vi "Main PC Station.vi"() -> ()   [LabVIEW 2015]
uses:
  ramki konfiguracyjne.ctl
  wyj manip.ctl
  wyj auto.ctl
  klapki.ctl
  szablon odometry_filtered_local.ctl
  QMH Fundamentals - Message Cluster.ctl
  CANFrameControl.ctl
  safety_ctl.ctl
  <vilib>/Utility/inputDevices.llb/closeJoystick.vi
  Gobal for ROS.vi
  Global GPS.vi
  <vilib>/MediaMongrels Ltd/WebSockets/WebSockets/WebSockets.lvlib
panel:
  out "szablon VELOCITIES 3":T1
  in  "szablon VELOCITIES 2":T1
  in  "Vlin multiply":dbl
  out "STEERING out":T2
  in  "STEERING":T2
  in  "LABVIEW AUTONOMY DATA":T3={"linear"=0.0, "angular"=0.0, "lin div"=1.0, "ang div"=1.0} {"angular" format="%#_13g"; "linear" format="%#_13g"}
  in  "LV/ROS":enum16{"LABVIEW", "ROS"}(ring)
  in  "szablon odometry/filtered/local":T4
  out "CMD_VEL out":T5
  in  "szablon ARM DRIVE":T6
  out "diody wyj":T7
  in  "szablon VELOCITIES":T1
  in  "klawiatura":bool
  in  "szukaj joy":bool=TRUE
  in  "wyszukaj\nxbox":bool=TRUE
  out "zakresy":cluster{"zak2":bool, "zak1":bool}
  out "MANIPULATOR wy 2":T8
  in  "path":path=path "C:/Users/Kacper/Desktop/Raptorv4/LOGI PREDKOSCI"
  in  "LOG?":bool
  out "RAW NAPEDY":T9
  in  "AUTO":bool
  in  "szablon CMD_VEL":T5
  in  "ster zadane":cluster{dbl, dbl}
  in  "TRIGGER":bool
  out "diody":T10
  in  "path to JPEG file":path=path "C:/Users/Kacper/Downloads/14331560_1175035659222212_341556152_n.png"
  in  "wlacz manipulator":bool
  out "kluster sterowan probnik":T11={"SERWO 6"=127, "SERWO 5"=127, "SERWO 4"=127, "SERWO 3"=127, "ON/OFF Wiertło"=FALSE, "Wiertło PWM"=128, "Wózek PWM"=128, "Stop głębokość"=TRUE, "Głębokość PWM"=128, "speed wózek"=0, "Wózek up"=FALSE, "Wózek down"=FALSE, "Stop wózek"=FALSE, "PROBNK ID 4"=3}
  in  "Zresetuj monitor":bool
  in  "Przestarzała data":bool
  in  "RESET STM":bool
  in  "STOP ??":bool
  out "speed out":cluster{i16, i16, i16, i16, i16, i16} {"?" scale=-32767.0..32767.0; "?" scale=-32767.0..32767.0; "?" scale=-32767.0..32767.0; "?" scale=-32767.0..32767.0; "?" scale=-32767.0..32767.0; "?" scale=-32767.0..32767.0}
  in  "E-Stop":bool
  out "srednie":T12(graph)
  out "UDP connection":bool
  in  "Tab Control 2":enum32{"CAN", "FPGA H&S", "SAFETY"}(tab)
  in  "Tab Control":T13(tab)
  out "Digital Waveform Graph":digitalwaveform(graph)
  out "Mixed Signal Graph":T14(graph)
  in  "STM Prawy ID CAN 2":u32=1
  in  "STM Lewy ID CAN 1":u32=2
  in  "IDD PREDKOSCI 1":u8=1
  in  "IDD PREDKOSCI  2":u8=1
  in  "PRZOD L":T15={"Prąd"=20.0, "Kp"=8.0, "Ki"=3.0, "OK Button"=FALSE, "ID CAN"=2, "IDD"=2, "Sat"=250} {"Ki" format="%.1f"; "Kp" format="%.1f"; "Prąd" format="%.1f"}
  in  "TYL L":T15={"Prąd"=20.0, "Kp"=8.0, "Ki"=3.0, "OK Button"=FALSE, "ID CAN"=2, "IDD"=3, "Sat"=250} {"Ki" format="%.1f"; "Kp" format="%.1f"; "Prąd" format="%.1f"}
  in  "SRODEK L":T15={"Prąd"=20.0, "Kp"=8.0, "Ki"=3.0, "OK Button"=FALSE, "ID CAN"=2, "IDD"=4, "Sat"=250} {"Ki" format="%.1f"; "Kp" format="%.1f"; "Prąd" format="%.1f"}
  in  "SRODEK P":T15={"Prąd"=20.0, "Kp"=8.0, "Ki"=3.0, "OK Button"=FALSE, "ID CAN"=1, "IDD"=4, "Sat"=250} {"Ki" format="%.1f"; "Kp" format="%.1f"; "Prąd" format="%.1f"}
  in  "TYL P":T15={"Prąd"=20.0, "Kp"=8.0, "Ki"=3.0, "OK Button"=FALSE, "ID CAN"=1, "IDD"=3, "Sat"=250} {"Ki" format="%.1f"; "Kp" format="%.1f"; "Prąd" format="%.1f"}
  in  "PRZOD P":T15={"Prąd"=20.0, "Kp"=8.0, "Ki"=3.0, "OK Button"=FALSE, "ID CAN"=1, "IDD"=2, "Sat"=250} {"Ki" format="%.1f"; "Kp" format="%.1f"; "Prąd" format="%.1f"}
  in  "wagi":T16={"l przod"=1.0, "l tyl"=1.0, "l srodek"=1.0, "p przod"=1.0, "p tyl"=1.0, "p srodek"=1.0} {"l przod" format="%#.6g"}
  in  "advertise msg":string="{\"op\":\"advertise\", \"topic\":\"pc/odom\",\"type\":\"sterowanie/velocities\"}"
  in  "rosbridge port":u16=9090
  in  "rosbridge server IP":string="192.168.1.117"
  in  "STOP ROS WRITE":bool
  out "raw frame":string
  in  "Topic to write":string="rio/odom"
  in  "ROSB WRITE":bool
  out "error out":errorcluster
  in  "ROSB READ":bool
  in  "stop 2":bool
  out "Opcode 2":u8
  out "Data 2":string
  in  "rosbridge server IP 2":string="192.168.164.128"
  in  "rosbridge port 2":u16=9090
  in  "error in (no error) 2":errorcluster
  out "error out 3":errorcluster
  in  "Topic to subscribe 2":string="/"
  out "Wykres manipulator":T17(graph)
  in  "Wej manip":T19={"MANIPULATOR ID 3 "=3, "0 bajt"=0, "serwa i pompa"={"4"=TRUE, "1 "=TRUE, "3"=TRUE, "2"=TRUE, "lewy"=TRUE, "serwo 3"=TRUE, "serwo 4 "=TRUE, "przekaznik"=TRUE}}
  in  "ster  manual manipulator":T20 {"DRUGIE 2" scale=0.0..255.0; "PIERWSZE 1" scale=0.0..255.0; "OBROT 0" scale=0.0..255.0; "OBROT 5" scale=0.0..255.0; "CHWYTAK 4" scale=0.0..255.0; "POCHYL 3" scale=0.0..255.0}
  in  "manual/wysylanie":bool
  out "MANIPULATOR wy":T17
  in  "Zbiornik 2":u8(slide)=128 scale=0.0..255.0
  in  "Stop zbiorniki 2":bool
  in  "Zbiornik":u8(slide)=128 scale=70.0..180.0
  in  "pojrmniki 6":u8(slide)=127 scale=0.0..255.0
  in  "SERWO 5":u8(slide)=127 scale=0.0..255.0
  in  "SERWO 4":u8(slide)=127 scale=0.0..255.0
  in  "chwytak 3":u8(slide)=127 scale=0.0..255.0
  in  "Stop głębokość":bool
  in  "Stop wózek":bool
  in  "Wiertło PWM":u8(slide)=128 scale=0.0..255.0
  in  "Gkebokość PWM":u8(slide)=128 scale=0.0..255.0
  in  "Wózek PWM":u8(slide)=128 caption="Vertical Pointer Slide" scale=0.0..255.0
  in  "ON/OFF Wiertło":bool
  in  "speed głębokość":u8
  in  "speed wózek":u8
  out "krańcówka 4":bool
  out "krańcówka 3":bool
  out "krańcówka 2":bool
  out "krańcówka":bool
  in  "PROBNK ID 4":u32=3
  in  "Wózek up":bool
  in  "Głębokość down":bool
  in  "Głębokość up":bool
  in  "Wózek down":bool
  in  "sterowanie joyem probe":bool
  in  "Stop zbiorniki":bool
  out "wiatr":T21 {"prędkosc wiatru km/h" scale=0.0..50.0}
  out "temp/wilg":T22
  out "zap/kierunek":T23
  out "pH":cluster{"temp. pkt rosy":sgl, "pH":sgl}
  in  "ROLL 1":dbl(slide) scale=0.0..1.0
  in  "YAW 1":dbl(slide) scale=0.0..1.0
  in  "PITCH 1":dbl(slide) scale=0.0..1.0
  in  "ile metrow ma przejechac ?":dbl=500.0
  out "teta":dbl
  out "Y":dbl
  out "X":dbl
  out "Location":cluster{"Y":dbl[], "Y":dbl[]}[](graph)
  in  "resset":bool
  in  "Xo":dbl
  in  "Yo":dbl=5.0
  in  "teta pocz.":dbl=90.0
  out "Yaw":dbl
  out "po korekcie":dbl
  out "pozycje z IMU":cluster{"Yaw":dbl, "Pitch":dbl, "Roll":dbl}(graph)
  in  "laser , obiekt ?":bool
  out "przejechane ?":bool
  out "obiekt?":bool
  in  "auto":T24={"zadany"=timestamp(0 s since 1904-01-01), "Autonomia ?"=FALSE, "Time Target (s)"=99999.0, "Reset"=FALSE, "odblokuj timer"=FALSE, "obiekt?"=FALSE, "przejechane ? "=FALSE} {"zadany" format="%<%H:%M:%S\n%x>T"}
  out "wyj auto":T25
  out "GPS Data":T26 {"Fix Quality" items=["Invalid", "GPS Fix", "DGPS Fix", "PPS Fix", "Real Time Kinematic", "Float RTK", "Estimated", "Manual Input Mode", "Simulation Mode"]}
  out "Frames":string[][](table)
  in  "Widocznosc ramek":bool=TRUE
  out "okres [ms]":dbl format="%.3g"
  out "ilosc mesagy":dbl
  in  "Prędkosci Prawy [4]":bool
  in  "Prędkości Lewy [5]":bool
  in  "manipulator [32]":bool
  out "wyj nowe L ?":cluster{"9":sgl, "10":sgl, "8":sgl}
  out "wyj nowe P ? 2":cluster{"9":sgl, "10":sgl, "8":sgl}
  in  "okres watchdoga":u32=100
  in  "wlacz watchdoga":bool
  out "temperatura":sgl(slide) scale=25.0..70.0
  in  "Total (%)":dbl(knob) scale=0.0..100.0
  in  "System Reset":bool
  out "kolejka odbior":i32
  out "kolejka wysylanie":i32
  in  "udp to sbrio":bool
  in  "eventy stop":bool
  out "send ind":i32
  in  "stop queue":bool
  out "receive ind":i32
  in  "UDP odbior in":bool
  in  "stop all":bool
  in  "UDP from sb 2":bool=TRUE
  in  "UDP to sb 2":bool=TRUE
  out "eventy ind":i32
  out "send loop":i32
  out "reciev lloop":i32
  out "safety":i32
  out "lok":i32
  out "lok1":i32
  out "jazda":i32
  out "mani":i32
  out "can":i32
  out "stope health":bool
  out "stope event":bool
  out "stope lokal":bool
  out "stope manip":bool
  out "stope jazda":bool
  out "stope lokal 2":bool
  out "stope odbior":bool
  out "stope wysyl":bool
  out "stope can":bool=TRUE
  out "# pending insert":i32
  out "# pending remove":i32
  in  "index joya\n jazda":i32
  in  "device index":i32=4
  out "wysylanie":bool
  out "graph drazki":cluster{i32[], i32[]}[](graph)
  out "ster. wyj. manipulator":T27
  out "Blokada jazda":bool
  out "graph 1":cluster{i32[], i32[]}[](graph)
  in  "max pwm skrecanie":dbl(slide)=0.5 scale=0.0..1.0
  in  "max pwm przod":dbl(slide)=0.5 min=0.0 max=255.0 scale=0.0..1.0
  out "Wysylanie jazda":bool
  # "max rotation +"
  # "max speed +"
  # "max rotation -"
  # "max speed -"
  # "Os Y +"
  # "Os X +"
  # "trigger"
  # "pitch grip"
  # "PWM 3 os Y\nPWM 4 os X\nPWM 5 T"
  # "gimbal 1"
  # "grip O/Z"
  # "gimbal 2"
  # "roll grip"
  # "Os Y+"
  # "ramie 1"
  # "PWM1 os X \nPWM2 os Y\nPWM 6 T"
  # "ramie 2"
  # "PWM 7 T"
  # "obrot base"
  # "Os X +"
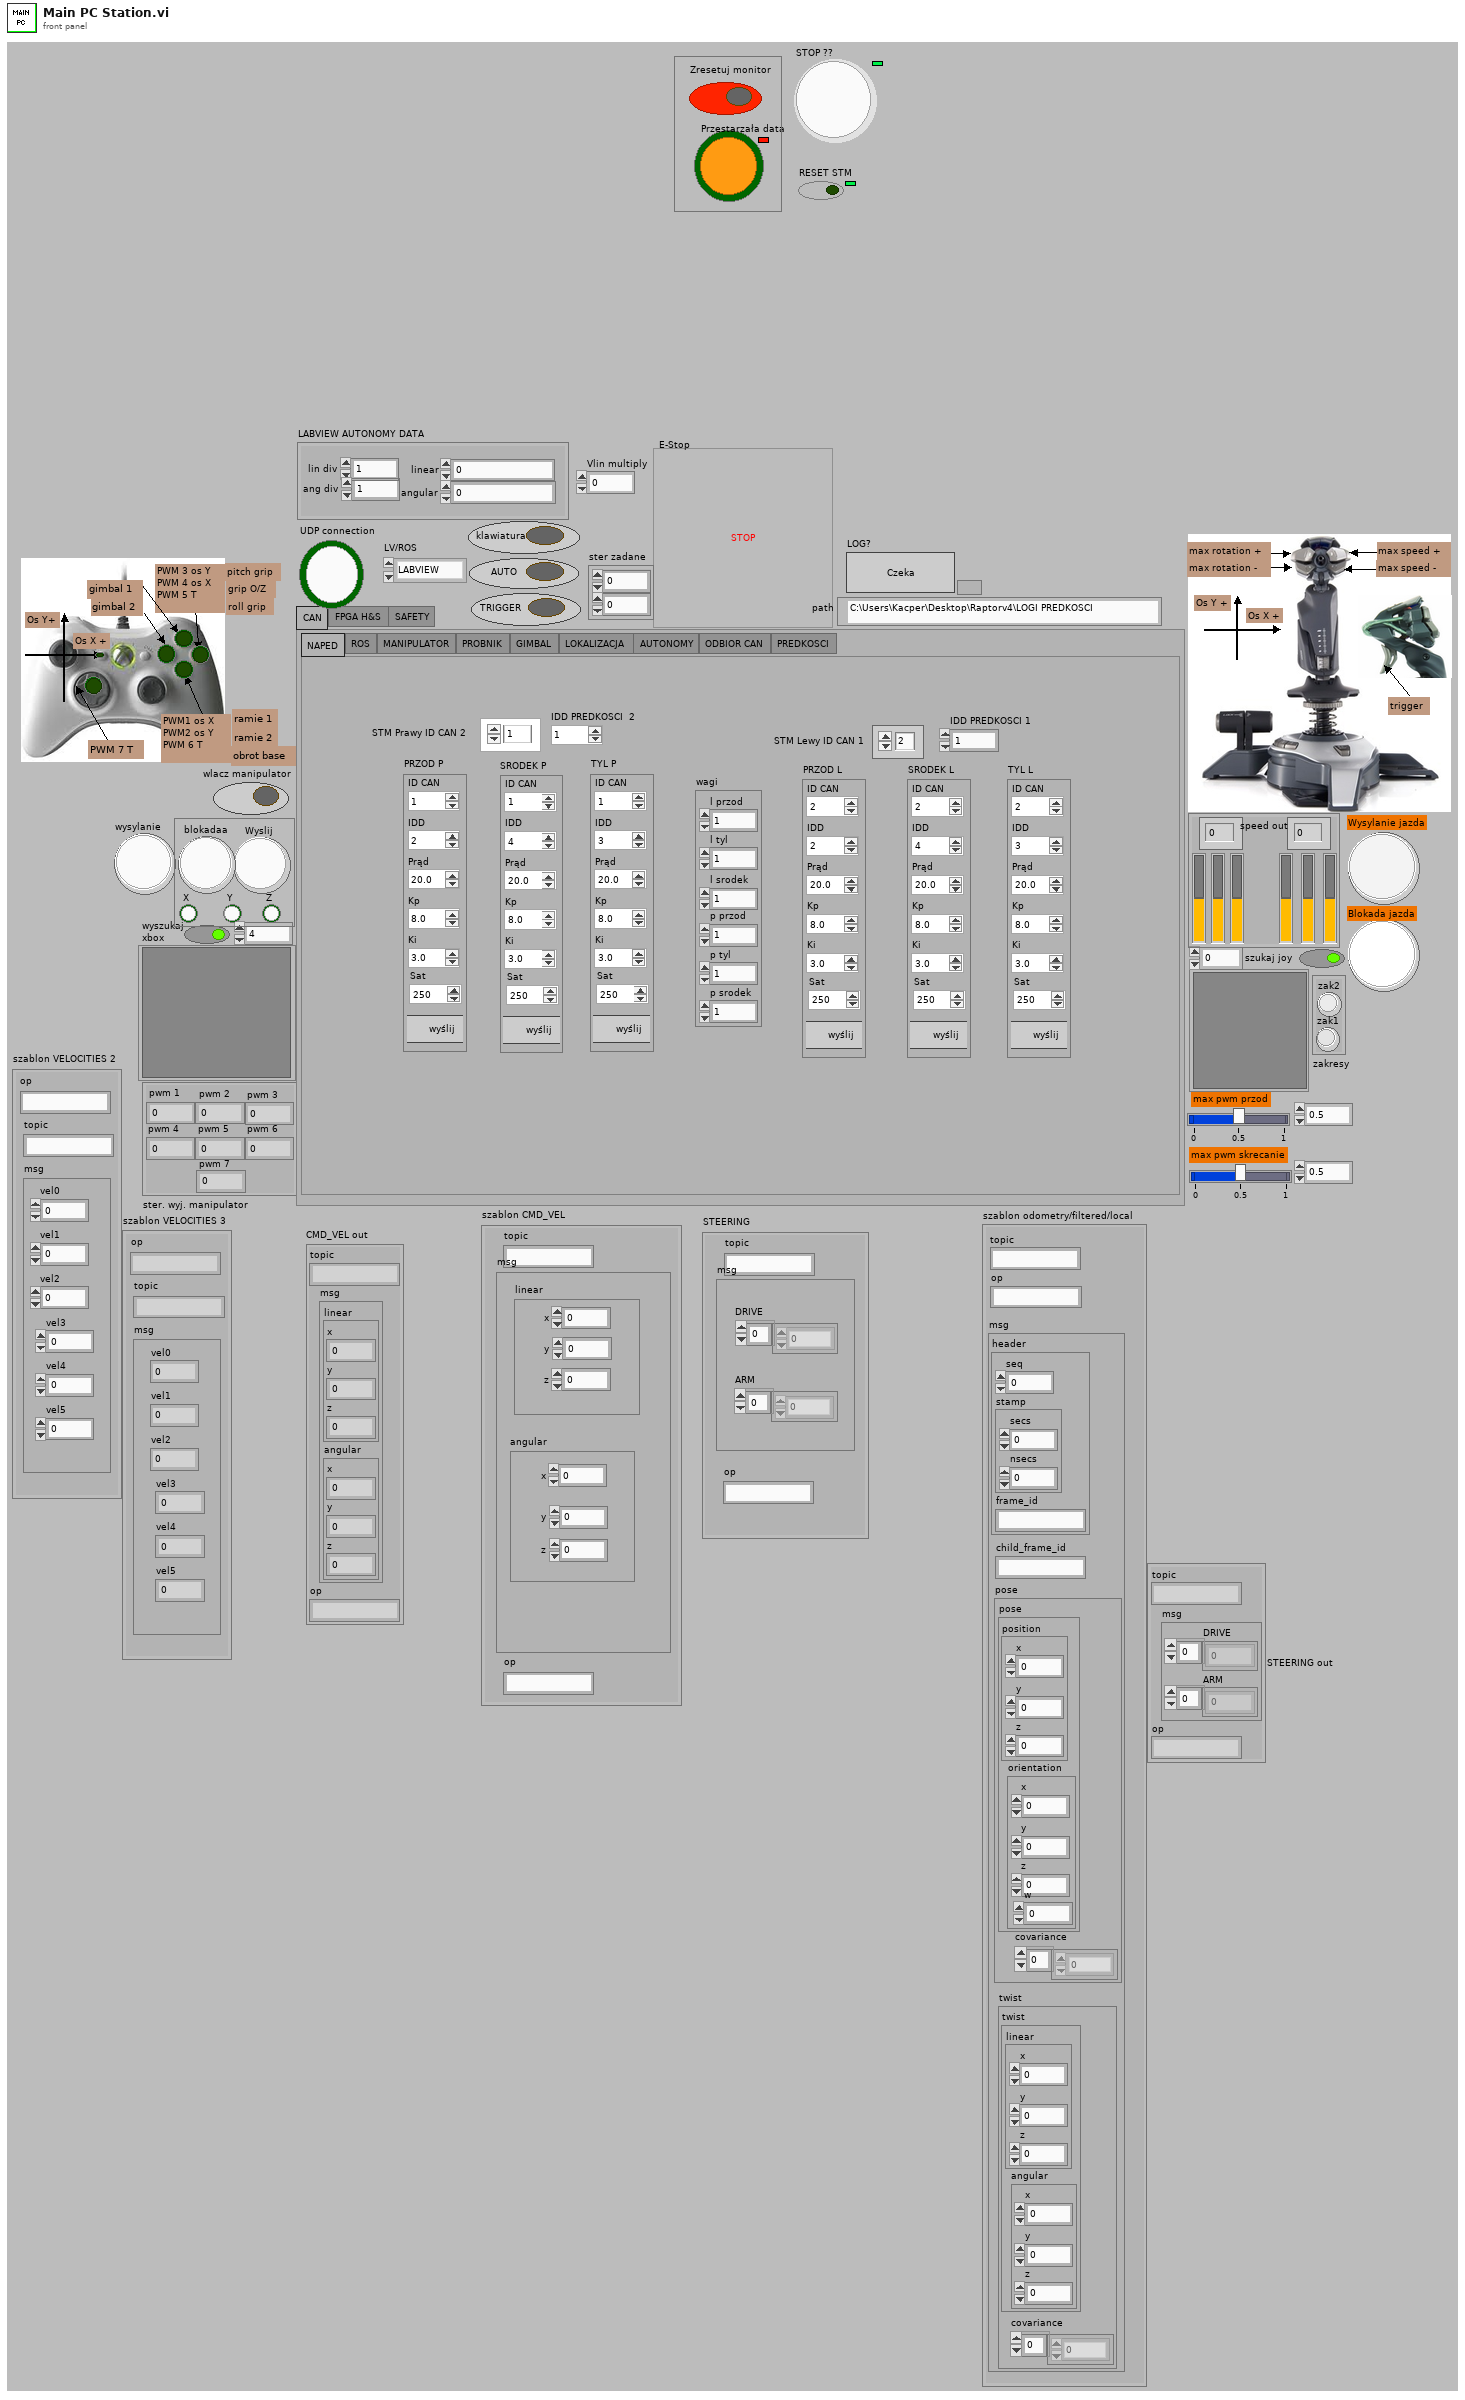
[diagram p1: front panel]
types:
  T1 = cluster{"op":string, "topic":string, "msg":cluster{"vel0":i16, "vel1":i16, "vel2":i16, "vel3":i16, "vel4":i16, "vel5":i16}}
  T2 = cluster{"topic":string, "msg":cluster{"DRIVE":i16[], "ARM":i8[]}, "op":string}
  T3 = cluster{"linear":dbl, "angular":dbl, "lin div":dbl, "ang div":dbl}
  T4 = typedef "szablon odometry_filtered_local.ctl" = cluster{"topic":string, "msg":cluster{"header":cluster{"seq":u32, "stamp":cluster{"secs":u32, "nsecs":i32}, "frame_id":string}, "child_frame_id":string, "pose":cluster{"pose":cluster{"position":cluster{"y":dbl, "z":dbl, "x":dbl}, "orientation":cluster{"y":dbl, "z":dbl, "x":dbl, "w":dbl}}, "covariance":dbl[]}, "twist":cluster{"twist":cluster{"linear":cluster{"y":dbl, "z":dbl, "x":dbl}, "angular":cluster{"y":dbl, "z":dbl, "x":dbl}}, "covariance":dbl[]}}, "op":string}
  T5 = cluster{"topic":string, "msg":cluster{"linear":cluster{"x":dbl, "y":dbl, "z":dbl}, "angular":cluster{"x":dbl, "y":dbl, "z":dbl}}, "op":string}
  T6 = cluster{"op":string, "topic":string, "msg":cluster{"DRIVE":i16[], "ARM":i8[]}}
  T7 = cluster{" X":bool, " Y":bool, " Z":bool, "blokadaa":bool, "Wyslij":bool}
  T8 = cluster{"bajt1":u8, "bajt2":u8, "bajt3":u8, "bajt4":u8, "bajt5":u8, "bajt6":u8, "bajt7":u8, "bajt8":u8}
  T9 = cluster{cluster{i16, i16, i16}, cluster{i16, i16, i16}}
  T10 = typedef "wyj manip.ctl" = cluster{"button 1":bool, "button 2":bool, "button 3":bool, "button 4":bool, "button 5":bool, "POV":bool}
  T11 = cluster{"SERWO 6":u8, "SERWO 5":u8, "SERWO 4":u8, "SERWO 3":u8, "ON/OFF Wiertło":bool, "Wiertło PWM":u8, "Wózek PWM":u8, "Stop głębokość":bool, "Głębokość PWM":u8, "speed wózek":u8, "Wózek up":bool, "Wózek down":bool, "Stop wózek":bool, "PROBNK ID 4":u32}
  T12 = cluster{"mean":dbl, "mean":dbl, "mean":dbl, "mean":dbl, "mean":dbl, "mean":dbl}
  T13 = enum32{"NAPED", "ROS", "MANIPULATOR", "PROBNIK", "GIMBAL", "LOKALIZACJA", "AUTONOMY", "ODBIOR CAN", "PREDKOSCI"}
  T14 = cluster{"digital waveform":digitalwaveform, u32[]}
  T15 = typedef "ramki konfiguracyjne.ctl" = cluster{"Prąd":dbl, "Kp":dbl, "Ki":dbl, "OK Button":bool, "ID CAN":u32, "IDD":u8, "Sat":u8}
  T16 = cluster{"l przod":dbl, "l tyl":dbl, "l srodek":dbl, "p przod":dbl, "p tyl":dbl, "p srodek":dbl}
  T17 = cluster{"bajt0":u8, "bajt1":u16, "bajt2":u16, "bajt3":u16, "bajt4":u16, "bajt5":u16, "bajt6":u8, "bajt7":u8}
  T18 = typedef "klapki.ctl" = cluster{"4":bool, "1 ":bool, "3":bool, "2":bool, "lewy":bool, "serwo 3":bool, "serwo 4 ":bool, "przekaznik":bool}
  T19 = cluster{"MANIPULATOR ID 3 ":u32, "0 bajt":u8, "serwa i pompa":T18}
  T20 = cluster{"OBROT 0":u8, "PIERWSZE 1":u8, "DRUGIE 2":u8, "POCHYL 3":u8, "CHWYTAK 4":u8, "OBROT 5":u8, "Numeric 6":i16}
  T21 = cluster{"pH":sgl, "metan":u8, "prędkosc wiatru km/h":u16, "kontaktron":u8}
  T22 = cluster{"temperatura 1 [C]":sgl, "wilgotnosc [%]":sgl}
  T23 = cluster{"zapylenie [ug/m^3] ":sgl, "kierunek wiatru [stopnie]":sgl}
  T24 = cluster{"zadany":timestamp, "Autonomia ?":bool, "Time Target (s)":dbl, "Reset":bool, "odblokuj timer":bool, "obiekt?":bool, "przejechane ? ":bool}
  T25 = typedef "wyj auto.ctl" = cluster{"AUTO ?":bool, "zadany czas":bool, "Time has Elapsed":bool, "Elapsed Time (s)":dbl, "seconds since 1Jan1904":timestamp}
  T26 = cluster{"Oldest Read Timestamp":timestamp, "Latitude":dbl, "Longitude":dbl, "Speed over Ground (Knots)":dbl, "True Track Angle (Deg)":dbl, "Altitude Above Mean Sea Level":dbl, "number of satellites in view.number of satellites":i8, "Fix Quality ":u16}
  T27 = cluster{"pwm 1":i16, "pwm 2":i16, "pwm 3":i16, "pwm 4":i16, "pwm 5":i16, "pwm 6":i16, "pwm 7":i16}
  T28 = typedef "QMH Fundamentals - Message Cluster.ctl" = cluster{"Message":string, "Message Data":variant}
  T29 = cluster{"queue out":refnum<queue>, "error out":errorcluster}
  T30 = typedef "CANFrameControl.ctl" = cluster{"identifier":u32, "extended?":bool, "type":u8, "payload":u8[]}
  T31 = typedef "Wyjscia joya.ctl" = cluster{"button 1":bool, "button 2":bool, "button 3":bool, "button 4":bool, "button 5":bool, "button 6":bool, "button 7":bool, "button 8":bool, "button 9":bool, "POV":bool, "button 10":bool}
  T32 = cluster{"X axis":i32, "Y axis":i32, "Z axis":i32, "X axis rotation":i32, "Y axis rotation":i32, "Z axis rotation":i32, "U axis":i32, "V axis":i32}
  T33 = cluster{"STM Lewy ID CAN 1":u32, "STM Prawy ID CAN 2":u32, "IDD PREDKOSCI 1":u8, "IDD PREDKOSCI  2":u8}
  T34 = cluster{"zakres X":bool, "zakres Y":bool, "zakres Z":bool, "blokadaa":bool, "Wyslij":bool}
  T35 = cluster{"CAN frame":T30, "GPS Data":cluster{"Oldest Read Timestamp":timestamp, "Latitude":dbl, "Longitude":dbl, "Speed over Ground (Knots)":dbl, "True Track Angle (Deg)":dbl, "Altitude Above Mean Sea Level":dbl, "number of satellites in view.number of satellites":i8, "Fix Quality ":u16}}
  T36 = cluster{cluster{"Decimal Number":sgl, "Decimal Number":sgl, "Decimal Number":sgl}, cluster{"Decimal Number":sgl, "Decimal Number":sgl, "Decimal Number":sgl}}
  T37 = cluster{"zap/kierunek":cluster{"zapylenie [ug/m^3] ":sgl, "kierunek wiatru [stopnie]":sgl}, "wiatr":cluster{"pH":sgl, "metan":u8, "prędkosc wiatru km/h":u16, "kontaktron":u8}, "temp/wilg":cluster{"temperatura 1 [C]":sgl, "wilgotnosc [%]":sgl}, "pH":cluster{"temp. pkt rosy":sgl, "pH":sgl}}
  T38 = cluster{"topic":string, "msg":cluster{"header":cluster{"seq":u32, "stamp":cluster{"secs":u32, "nsecs":i32}, "frame_id":string}, "buttons":i32[], "axes":sgl[]}, "op":string}
  T39 = cluster{"header":cluster{"seq":u32, "stamp":cluster{"secs":u32, "nsecs":i32}, "frame_id":string}, "buttons":i32[], "axes":sgl[]}
  T40 = typedef "imagedata.ctl" = cluster{"image type":i32, "image depth":i32, "image":u8[], "mask":u8[], "colors":u32[], "Rectangle":cluster{"left":i16, "top":i16, "right":i16, "bottom":i16}}
  T41 = cluster{"port wysyłania":u16, u32, "port":refnum<k16>, "error out":errorcluster}
  T42 = cluster{"Queue in":refnum<queue>, "error out":errorcluster}
  T43 = cluster{"PITCH 1":dbl, "YAW 1":dbl, "ROLL 1":dbl}
  T44 = typedef "safety_ctl.ctl" = cluster{"reset_stm":bool, "stop":bool}
  T45 = typedef "eventvkey.ctl" = enum16{"ASCII", "Enter", "Return", "Shift", "Ctrl", "Alt", "Cmd", "Opt", "Caps", "NumLock", "Clear", "Break", "Up", "Down", "Left", "Right", "Insert", "Delete", "Home", "End", "PageUp", "PageDown", "Escape", "Help", "Pause", "ScrollLock", "F1", "F2", "F3", "F4", "F5", "F6", "F7", "F8", "F9", "F10", "F11", "F12", "F13", "F14", "F15", "F16", "F17", "F18", "F19", "F20", "F21", "F22", "F23", "F24", "Play", "VolumeUp", "VolumeDown", "Mute", "Two Byte Char"}
  T46 = cluster{"pojrmniki 6":u8, "SERWO 5":u8, "SERWO 4":u8, "chwytak 3":u8, "ON/OFF Wiertło":bool, "Wiertło PWM":u8, "Gkebokość PWM":u8, "Stop głębokość":bool, "Wózek PWM":u8, "speed wózek":u8, "Wózek up":bool, "Wózek down":bool, "Stop wózek":bool, "PROBNK ID 4":u32}
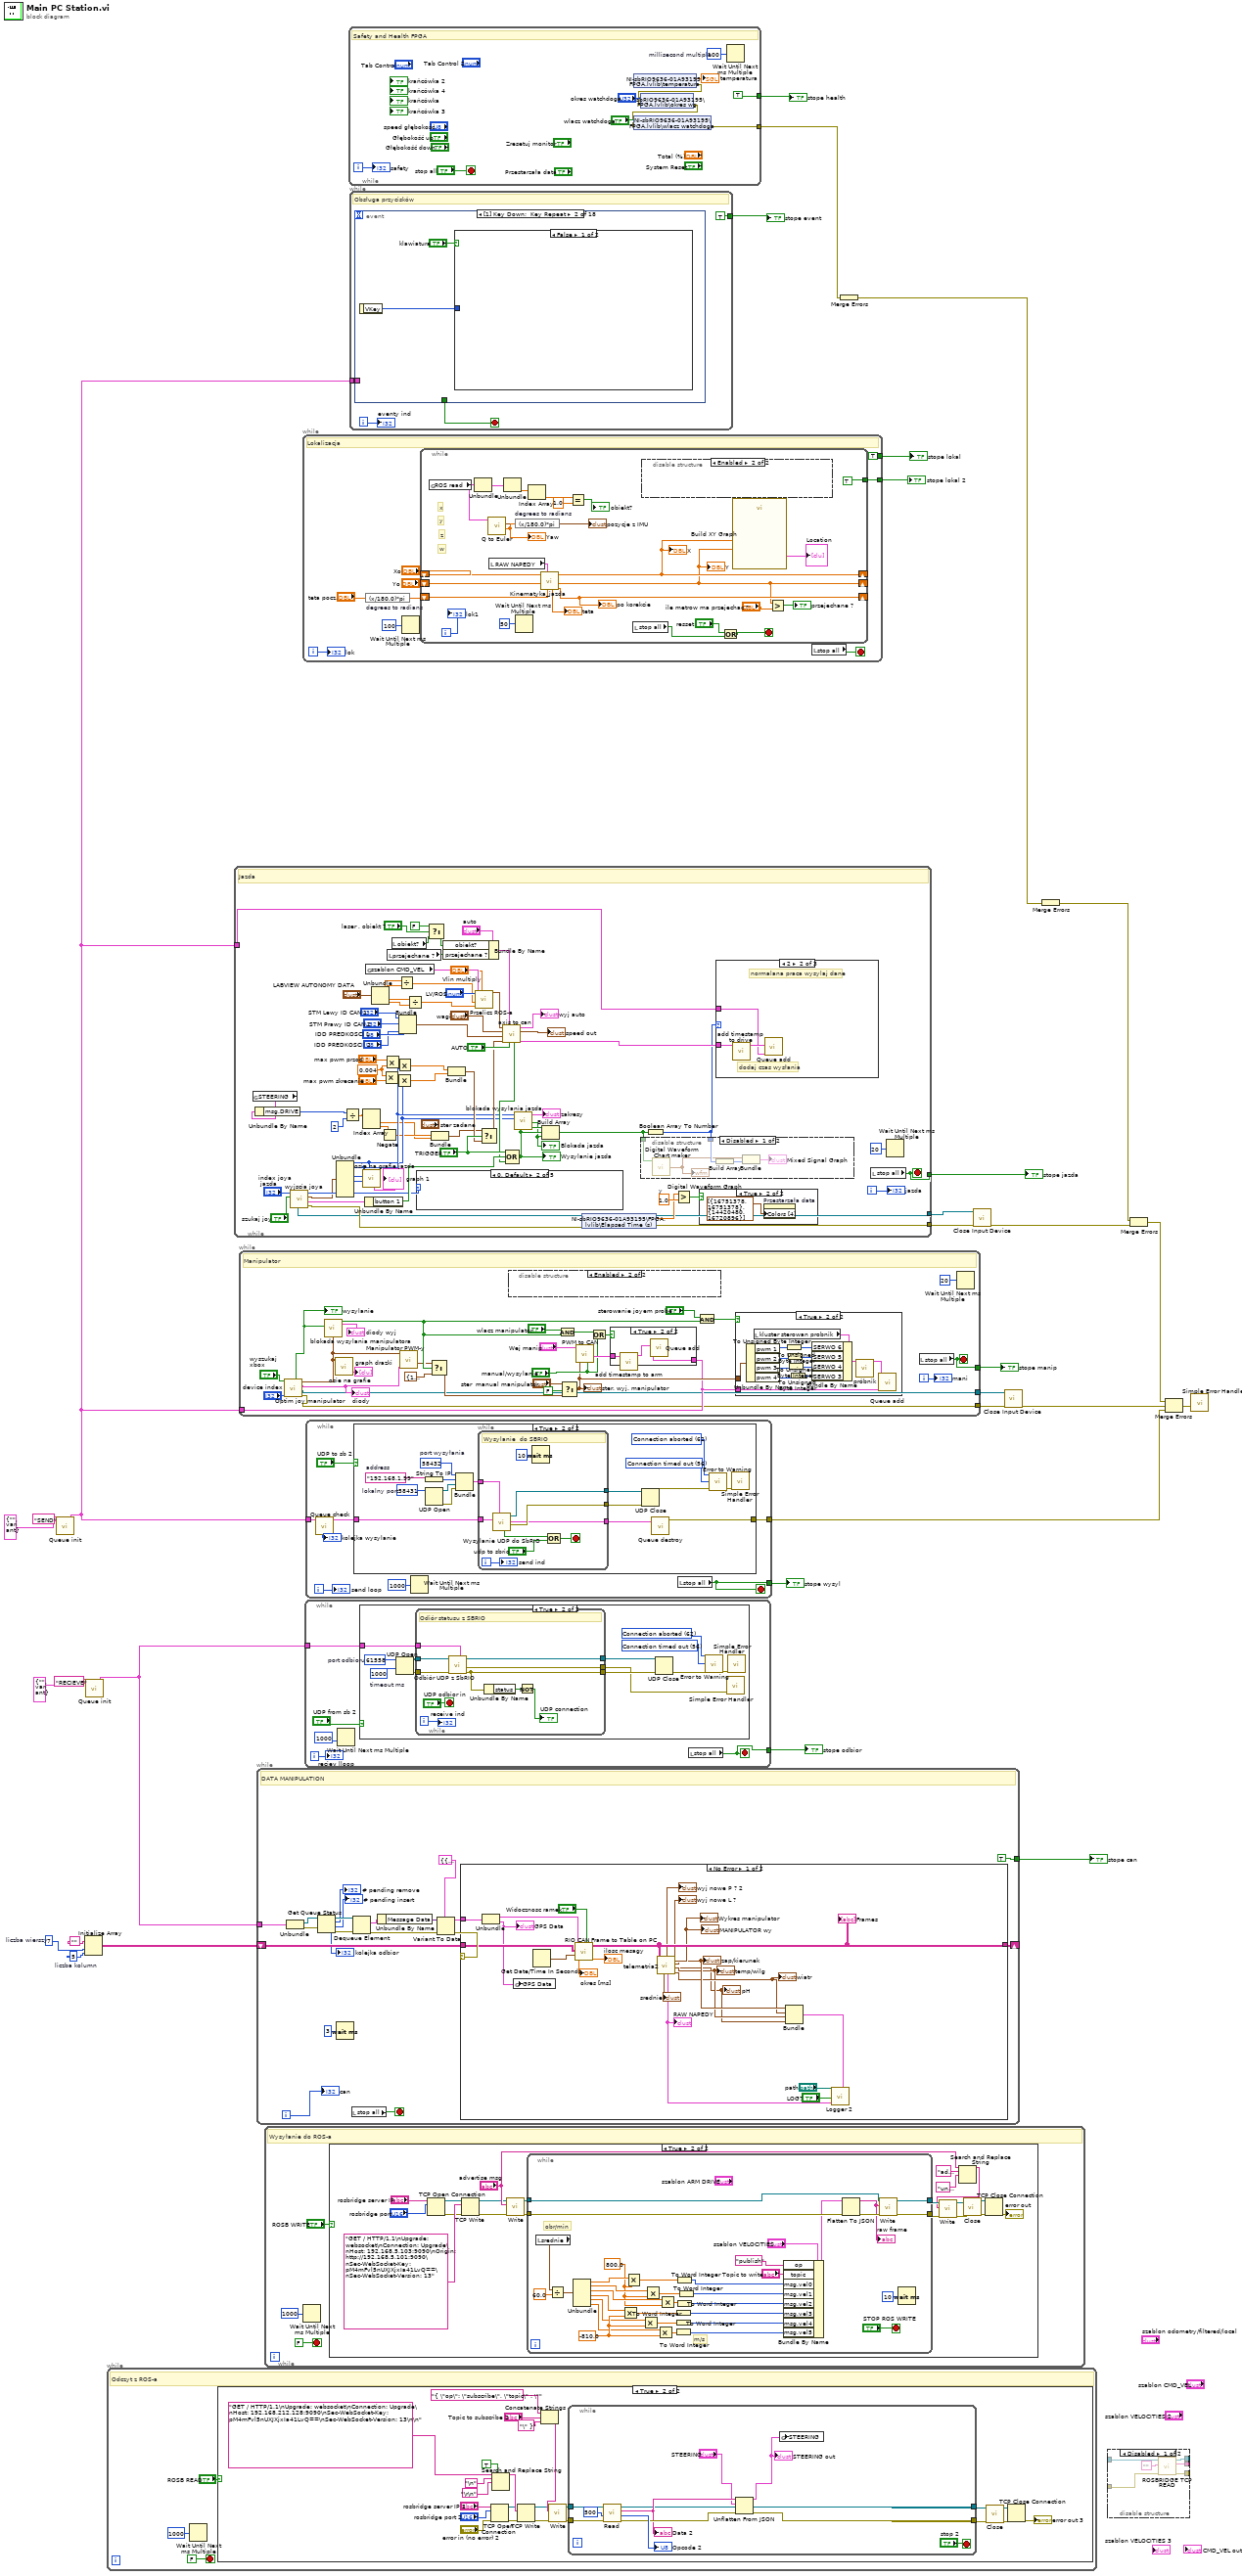
[diagram p0: block diagram]
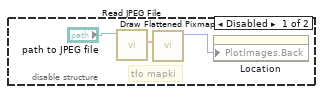
[diagram p5: hidden frame]
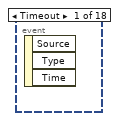
[diagram p7: hidden frame]
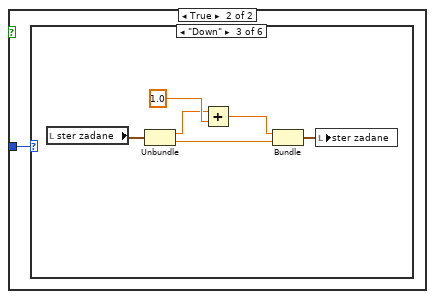
[diagram p8: hidden frame]
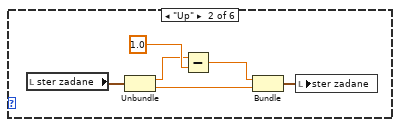
[diagram p10: hidden frame]
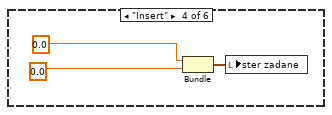
[diagram p11: hidden frame]
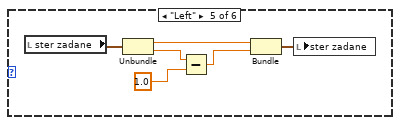
[diagram p12: hidden frame]
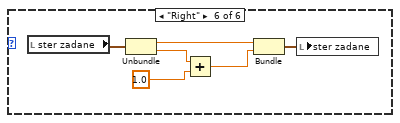
[diagram p13: hidden frame]
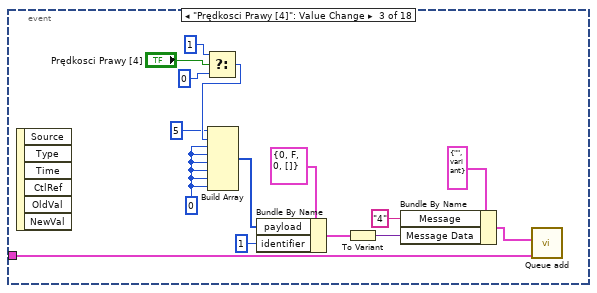
[diagram p14: hidden frame]
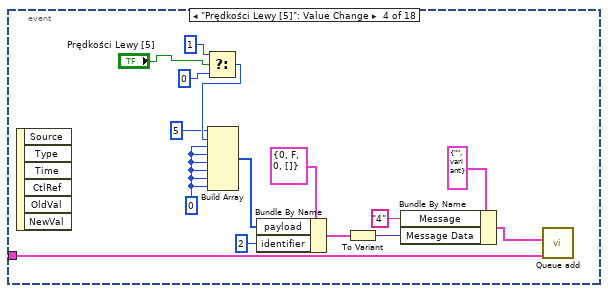
[diagram p15: hidden frame]
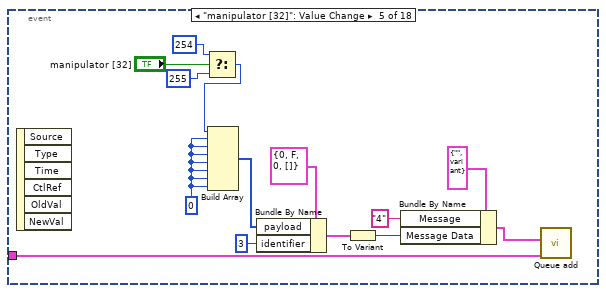
[diagram p16: hidden frame]
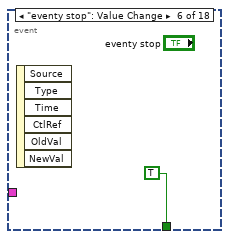
[diagram p17: hidden frame]
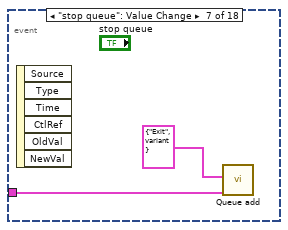
[diagram p18: hidden frame]
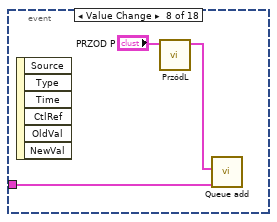
[diagram p19: hidden frame]
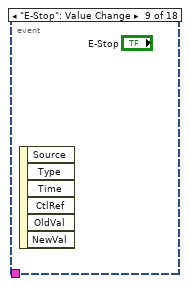
[diagram p20: hidden frame]
diagram:
  w24 = 7  # liczba wierszy
  w23 = 5  # liczba kolumn
  n1 = call "Queue init.vi"("Message Cluster"=T28 {"Message"="", "Message Data"=variant}, "name (unnamed)"="SEND") -> ("Cluster"=w4:T29)  [unwired: 9 in]
  n2 = Initialize Array("" ("Empty String Constant"), w24, w23) -> (w21:string[][])
  n3 = call "Queue init.vi"("Message Cluster"=T28 {"Message"="", "Message Data"=variant}, "name (unnamed)"="RECIEVE") -> ("Cluster"=w1:T29)  [unwired: 9 in]
  n4 = while {
    stop <- FALSE stop-if-true
    # "Odczyt z ROS-a"
    n5 = Wait Until Next ms Multiple(millisecond multiple=u32 1000 ("milliseconds to wait")) -> ()  [unwired: 1 out]
    n6 = case shown="True" "ROSB READ" {
      frame False {
      }
      frame True {
        n7 = TCP Open Connection(address="rosbridge server IP 2", remote port or service name="rosbridge port 2", error in (no error)="error in (no error) 2") -> (connection ID=w37:refnum<k5>, error out=w38:errorcluster)  [unwired: 2 in]
        n8 = Search and Replace String(replace all?=TRUE ("replace all? (F)"), input string="GET / HTTP/1.1\nUpgrade: websocket\nConnection: Upgrade\nHost: 192.168.212.128:9090\nSec-WebSocket-Key: pM4mFvl5nUXJXjxIa41LvQ==\nSec-WebSocket-Version: 13\n\n", search string="\n", replace string="\r\n") -> (result string=w53:string)  [unwired: 4 in, 3 out]
        n9 = TCP Write(connection ID=w37, data in=w53, error in (no error)=w38) -> (connection ID out=w41:refnum<k5>, error out=w42:errorcluster)  [unwired: 1 in, 1 out]
        n10 = Concatenate Strings("{ \"op\": \"subscribe\", \"topic\" : \"", "Topic to subscribe 2", "\" }") -> (w55:string)
        n11 = call <vilib>:"Write.vi"("error in (no error)"=w42, "Data"=w55, "WebSocket Connection in"=w41) -> ("error out"=w46:errorcluster, "WebSocket Connection out"=w45:refnum<k5>)  [unwired: 7 in]
        n12 = while {
          tunnel: [w61] -> w43
          tunnel: [w60] -> w44
          tunnel: w45 -> [w68]
          tunnel: w46 -> [w67]
          stop <- "stop 2" stop-if-true
          n13 = call <vilib>:"Read.vi"("error in (no error)"=w67, "timeout ms (5000)"=500, "WebSocket Connection in"=w68) -> ("error out"=w64:errorcluster, "Opcode"=→"Opcode 2":u8, "Data"=w63:string, "WebSocket Connection out"=w61:refnum<k5>)  [unwired: 5 in]
          "Data 2" <- w63
          n14 = Unflatten From JSON(JSON string=w63, type and defaults="STEERING", error in (no error)=w64) -> (value=w58:T2, error out=w60:errorcluster)  [unwired: 4 in]
          "STEERING out" <- w58
          n15 = global write "Gobal for ROS.vi" "STEERING"(w58) -> ()
        }
        n16 = call <vilib>:"Close.vi"("error in (no error)"=w44, "WebSocket Connection in"=w43) -> ("error out"=w40:errorcluster, "WebSocket Connection in"=w39:refnum<k5>)  [unwired: 8 in]
        n17 = TCP Close Connection(connection ID=w39, error in (no error)=w40) -> (error out=→"error out 3":errorcluster)  [unwired: 1 in, 1 out]
      }
    }
  }
  n18 = while {
    tunnel: [w88] -> w31
    tunnel: [w128] -> w30
    tunnel: [w103] -> w17
    tunnel: w4 -> [w95]
    i -> [w114]
    stop <- w103 stop-if-true
    w109 = 0.004 ("y")
    w131 = 1.0  # y
    # "Jazda"
    n19 = global read "Gobal for ROS.vi" "STEERING"() -> (w69:T2)
    n20 = Unbundle By Name(w69) -> ("msg.DRIVE"=w75:i16[])
    n21 = call "wyjscia joya.vi"("szukaj joy"="szukaj joy", "index joya jazda"="index joya\n jazda") -> ("error out"=w89:errorcluster, "wyjscia joya"=w90:T31, "axis info"=w91:T32, "number"=w92:u32, "Refnum out"=w88:refnum<k1>)  [unwired: 3 in]
    n22 = Unbundle(w91) -> ("X axis"=w78:i32, "Y axis"=w79:i32, "X axis rotation"=w139:i32, "Y axis rotation"=w140:i32)  [unwired: 4 out]
    n23 = Divide(x=w75, y=i16 2) -> (x/y=w77:dbl[])
    n24 = Index Array(array=w77) -> (element #1=w70:dbl, element #2=w72:dbl)  [unwired: 2 in]
    n25 = call "osie na grafie jazda.vi"("Y axis rotation"=w140, "X axis rotation"=w139, "Y axis"=w79, "X axis"=w78) -> ("graph 1"=→"graph 1":cluster{i32[], i32[]}[])  [unwired: 7 in]
    n26 = Unbundle By Name(w90) -> ("button 1"=w141:bool)
    n27 = global read "Gobal for ROS.vi" "szablon CMD_VEL"() -> (w105:T5)
    n28 = Unbundle("LABVIEW AUTONOMY DATA") -> ("linear"=w83:dbl, "angular"=w82:dbl, "lin div"=w81:dbl, "ang div"=w80:dbl)
    n29 = Negate(x=w72) -> (-x=w71:dbl)
    n30 = Multiply(x=w109, y="max pwm skrecanie") -> (x*y=w112:dbl)
    n31 = Multiply(x="max pwm przod", y=w109) -> (x*y=w108:dbl)
    n32 = local read "przejechane ?"() -> (w125:bool)
    n33 = local read "obiekt?"() -> (w123:bool)
    n34 = Multiply(x=w112, y=w78) -> (x*y=w113:dbl)
    n35 = Multiply(x=w108, y=w79) -> (x*y=w132:dbl)
    n36 = Divide(x=w83, y=w81) -> (x/y=w85:dbl)
    n37 = Bundle("STM Lewy ID CAN 1"="STM Lewy ID CAN 1", "STM Prawy ID CAN 2"="STM Prawy ID CAN 2", "IDD PREDKOSCI 1"="IDD PREDKOSCI 1", "IDD PREDKOSCI  2"="IDD PREDKOSCI  2") -> (w96:T33)  [unwired: 1 in]
    n38 = Divide(x=w82, y=w80) -> (x/y=w86:dbl)
    n39 = case shown="0, Default" w92 {
      frame 8 {
        n40 = local read "max pwm skrecanie"() -> (w162:dbl)
        n41 = Add(x=w162, y=0.01) -> (x+y=w158:dbl)
        n42 = In Range and Coerce(upper limit=1.0, x=w158, lower limit=0.0) -> (coerced(x)=w157:dbl)  [unwired: 1 out]
        n43 = local write "max pwm skrecanie"(w157) -> ()
      }
      frame 0, Default {
      }
      frame 1 {
        n44 = local read "max pwm przod"() -> (w163:dbl)
        n45 = Add(x=w163, y=0.01) -> (x+y=w164:dbl)
        n46 = In Range and Coerce(upper limit=1.0, x=w164, lower limit=0.0) -> (coerced(x)=w165:dbl)  [unwired: 1 out]
        n47 = local write "max pwm przod"(w165) -> ()
      }
      frame 2 {
        n48 = local read "max pwm przod"() -> (w169:dbl)
        n49 = Subtract(x=w169, y=0.01) -> (x-y=w170:dbl)
        n50 = In Range and Coerce(upper limit=1.0, x=w170, lower limit=0.0) -> (coerced(x)=w171:dbl)  [unwired: 1 out]
        n51 = local write "max pwm przod"(w171) -> ()
      }
      frame 4 {
        n52 = local read "max pwm skrecanie"() -> (w180:dbl)
        n53 = Subtract(x=w180, y=0.01) -> (x-y=w177:dbl)
        n54 = In Range and Coerce(upper limit=1.0, x=w177, lower limit=0.0) -> (coerced(x)=w178:dbl)  [unwired: 1 out]
        n55 = local write "max pwm skrecanie"(w178) -> ()
      }
    }
    n56 = Select(t=FALSE, s="laser , obiekt ?", f=w123) -> (s? t:f=w124:bool)
    n57 = Bundle(w71, w70) -> (w73:cluster{dbl, dbl})  [unwired: 1 in]
    n58 = Bundle By Name(cluster="auto", "obiekt?"=w124, "przejechane ?"=w125) -> (w126:T24)
    n59 = Bundle(w132, w113) -> (w106:cluster{dbl, dbl})  [unwired: 1 in]
    n60 = call "Przelicz ROS-a.vi"("Vlin multiply"="Vlin multiply", "angular"=w86, "linear"=w85, "Enum"="LV/ROS", "szablon CMD_VEL"=w105) -> ("ROS data converted"=w98:cluster{dbl, dbl})  [unwired: 6 in]
    n61 = Select(t=w73, s="TRIGGER", f=w106) -> (s? t:f=w97:cluster{dbl, dbl})
    n62 = call "axis to can.vi"("ROS"="AUTO", "wej auto"=w126, "wej ster"=w97, "wej  ID"=w96, "wej wagi"="wagi", "ROS in"=w98) -> ("array of cans"=w138:T30[], "wyj pred"=→"speed out":cluster{i16, i16, i16, i16, i16, i16}, "wyj auto"=→"wyj auto":T25, "wyślij"=w99:bool)  [unwired: 2 in]
    n63 = Compound Arithmetic op=OR("TRIGGER", w141, w99) -> (w117:bool)
    "Wysylanie jazda" <- w117
    n64 = call "blokada wysylania jazda.vi"("wysylanie"=w117, "X axis"=w78, "Y axis"=w79) -> ("fall edge wysl"=w120:bool, "blokada jazdy"=w100:bool, "zakresy"=→"zakresy":cluster{"zak2":bool, "zak1":bool})  [unwired: 6 in]
    "Blokada jazda" <- w100
    n65 = Build Array(w120, w117, w100) -> (w119:bool[])
    n66 = shared-variable "NI-sbRIO9636-01A93195\\FPGA.lvlib\\Elapsed Time (s)"(error in=w89) -> (w129:dbl, error out=w128:errorcluster)
    n67 = Boolean Array To Number(Boolean array=w119) -> (number=w118:u32)
    n68 = disable-structure shown="Disabled" {
      disable-tunnel: w119 -> [w147 _]
      disable-tunnel: w118 -> [w146 _]
      frame Disabled {
        n69 = call "Digital Waveform Chart maker.vi"("Array"=w147) -> ("digital waveform"=w145:digitalwaveform)  [unwired: 3 in]
        "Digital Waveform Graph" <- w145
        n70 = Build Array(w146) -> (w144:u32[])
        n71 = Bundle("digital waveform"=w145, w144) -> (→"Mixed Signal Graph":T14)  [unwired: 1 in]
      }
      frame Enabled {
      }
    }
    n72 = Greater?(x=w129, y=w131) -> (0:w130:bool)
    n73 = case shown="True" w130 {
      frame False {
      }
      frame True {
        n74 = property on="Przestarzała data" class="Bool (strict)"("Colors [4]"=cluster{u32, u32}[] [{16751378, 16751378}, {14420480, 16720896}]) -> ()  [unwired: 2 in, 2 out]
      }
    }
    n75 = case shown="2" w118 {
      tunnel: w138 -> [_ w151 _]
      tunnel: w95 -> [_ w149 w152]
      frame 0, Default {
      }
      frame 2 {
        # "dodaj czas wysłania"
        # "normalana praca wysylaj dane"
        n76 = call "add timestamp to drive.vi"("array of cans"=w151) -> ("Message Cluster"=w150:T28)  [unwired: 10 in]
        n77 = call "Queue add.vi"("Queue B in"=w149, "Message Cluster"=w150) -> ()  [unwired: 10 in]
      }
      frame 1 {
        # "dla zbocza opadajacego  wyslij predkosci zerowe"
        n78 = for {
          N: 3 -> [_]
          tunnel: w152 -> [w156]
          n79 = call "add timestamp to drive.vi"("array of cans"=T30[] [{"identifier"=1, "extended?"=FALSE, "type"=0, "payload"=[1, 0, 0, 0, 0, 0, 0, 0]}, {"identifier"=2, "extended?"=FALSE, "type"=0, "payload"=[1, 0, 0, 0, 0, 0, 0, 0]}] ("zerowanie predkosci")) -> ("Message Cluster"=w154:T28)  [unwired: 10 in]
          n80 = call "Queue add.vi"("Queue B in"=w156, "Message Cluster"=w154) -> ()  [unwired: 10 in]
        }
      }
    }
    n81 = local read "stop all"() -> (w103:bool)
    n82 = Wait Until Next ms Multiple(millisecond multiple=i16 20 ("milliseconds to wait")) -> ()  [unwired: 1 out]
    "jazda" <- w114
  }
  "stope jazda" <- w17
  n83 = while {
    tunnel: [w183] -> w29
    tunnel: [w182] -> w28
    tunnel: [w195] -> w16
    tunnel: w4 -> [w197]
    i -> [w203]
    stop <- w195 stop-if-true
    # "Manipulator"
    n84 = call "Optim joy manipulator.vi"("device index"="device index", "wyszukaj xbox"="wyszukaj\nxbox") -> ("error out"=w182:errorcluster, "Refnum out"=w183:refnum<k1>, "output cluster"=w184:T10, "axis info"=w185:T32, "wysylanie"=w186:bool)  [unwired: 5 in]
    "wysylanie" <- w186
    "diody" <- w184
    n85 = call "blokada wysylania manipulatora.vi"("axis info"=w185, "wysylanie"=w186) -> ("Wyslij"=w192:bool, "output cluster"=→"diody wyj":T34)  [unwired: 4 in, 4 out]
    n86 = call "osie na grafie.vi"("axis info"=w185) -> ("graph 2"=→"graph drazki":cluster{i32[], i32[]}[])  [unwired: 10 in]
    n87 = call "Manipulator PWM-y.vi"("output cluster"=w184, "axis info"=w185) -> ("wyj pwm manip."=w190:T27)  [unwired: 9 in]
    n88 = Select(t=w190, s=w192, f=T27 {"pwm 1"=127, "pwm 2"=127, "pwm 3"=127, "pwm 4"=127, "pwm 5"=127, "pwm 6"=127, "pwm 7"=127} ("output cluster")) -> (s? t:f=w189:T27)
    n89 = disable-structure shown="Enabled" {
      frame Disabled {
        n90 = local read item#-1() -> (w209)
        n91 = call "MANIPULATOR STER PID.vi"("MANIPULATOR wy 3"=w209) -> ("MANIPULATOR wy 2"=→"MANIPULATOR wy 2":T8)  [unwired: 10 in]
      }
      frame Enabled {
      }
    }
    n92 = And(x="wlacz manipulator", y=w192) -> (x .and. y?=w201:bool)
    n93 = Select(t="ster  manual manipulator", s=FALSE, f=w189) -> (s? t:f=w198:T27)
    "ster. wyj. manipulator" <- w198
    n94 = call "PWM to CAN.vi"("manual/wysylanie"="manual/wysylanie", "cluster manipulator 2"=w198, "Cluster"="Wej manip") -> ("array of cans"=w207:T30[])  [unwired: 6 in, 2 out]
    n95 = Or(x=w201, y="manual/wysylanie") -> (x .or. y?=w202:bool)
    n96 = case shown="True" w202 {
      tunnel: w207 -> [_ w225]
      tunnel: w197 -> [_ w226]
      frame False {
      }
      frame True {
        n97 = call "add timestamp to arm.vi"("array of cans"=w225) -> ("Message Cluster"=w224:T28)  [unwired: 10 in]
        n98 = call "Queue add.vi"("Queue B in"=w226, "Message Cluster"=w224) -> ()  [unwired: 10 in]
      }
    }
    n99 = And(x="sterowanie joyem probe", y=w192) -> (x .and. y?=w205:bool)
    n100 = case shown="True" w205 {
      tunnel: w198 -> [_ w211]
      tunnel: w197 -> [_ w212]
      frame False {
      }
      frame True {
        n101 = Unbundle By Name(w211) -> ("pwm 1"=w217:i16, "pwm 2"=w216:i16, "pwm 3"=w215:i16, "pwm 4"=w214:i16)
        n102 = local read "kluster sterowan probnik"() -> (w223:T11)
        n103 = To Unsigned Byte Integer(number=w217) -> (unsigned 8bit integer=w218:u8)
        n104 = To Unsigned Byte Integer(number=w216) -> (unsigned 8bit integer=w219:u8)
        n105 = To Unsigned Byte Integer(number=w215) -> (unsigned 8bit integer=w220:u8)
        n106 = To Unsigned Byte Integer(number=w214) -> (unsigned 8bit integer=w221:u8)
        n107 = Bundle By Name(cluster=w223, "SERWO 6"=w218, "SERWO 5"=w219, "SERWO 4"=w220, "SERWO 3"=w221) -> (w222:T11)
        n108 = call "próbnik.vi"("output cluster 2"=w222) -> ("Message Cluster"=w213:T28)  [unwired: 9 in, 1 out]
        n109 = call "Queue add.vi"("Queue B in"=w212, "Message Cluster"=w213) -> ()  [unwired: 10 in]
      }
    }
    n110 = local read "stop all"() -> (w195:bool)
    n111 = Wait Until Next ms Multiple(millisecond multiple=u32 20 ("milliseconds to wait")) -> ()  [unwired: 1 out]
    "mani" <- w203
  }
  "stope manip" <- w16
  n112 = while {
    shift-right: [w243] -> _
    shift-left: w21 -> [w246]
    tunnel: [TRUE] -> w12
    tunnel: w1 -> [w235]
    i -> [w244]
    stop <- w245 stop-if-true
    # "DATA MANIPULATION"
    n113 = Unbundle(w235) -> ("queue out"=w236:refnum<queue>, "error out"=w232:errorcluster)
    n114 = Get Queue Status(queue=w236, error in (no error)=w232) -> (queue out=w233:refnum<queue>, # pending remove=→"# pending remove":i32, # pending insert=→"# pending insert":i32, error out=w231:errorcluster, # elements in queue=→"kolejka odbior":i32)  [unwired: 1 in, 3 out]
    n115 = Wait (ms)(milliseconds to wait=u32 3) -> ()  [unwired: 1 out]
    n116 = local read "stop all"() -> (w245:bool)
    n117 = Dequeue Element(queue=w233, error in (no error)=w231) -> (element=w238:T28, error out=w237:errorcluster)  [unwired: 1 in, 2 out]
    n118 = Unbundle By Name(w238) -> ("Message Data"=w242:variant)
    n119 = Variant To Data(error in=w237, type=T35 {"CAN frame"={"identifier"=0, "extended?"=FALSE, "type"=0, "payload"=[]}, "GPS Data"={"Oldest Read Timestamp"=timestamp(0 s since 1904-01-01), "Latitude"=0.0, "Longitude"=0.0, "Speed over Ground (Knots)"=0.0, "True Track Angle (Deg)"=0.0, "Altitude Above Mean Sea Level"=0.0, "number of satellites in view.number of satellites"=0, "Fix Quality "=0}} ("output cluster"), Variant=w242) -> (data=w241:T35, error out=w240:errorcluster)
    n120 = case shown="No Error" w240 {
      tunnel: w246 -> [w267 w268]
      tunnel: [w266 w268] -> w243
      tunnel: w241 -> [w262 _]
      frame No Error {
        n121 = Unbundle(w262) -> ("CAN frame"=w261:T30, "GPS Data"=w256:T26)
        "GPS Data" <- w256
        n122 = global write "Global GPS.vi" "GPS Data"(w256) -> ()
        n123 = Get Date/Time In Seconds() -> (seconds since 1Jan1904=w258:timestamp)
        n124 = call "RIO CAN Frame to Table on PC.vi"("Widok ramek"="Widocznosc ramek", "timestamp"=w258, "Input CAN Array"=w267, "CAN frame"=w261) -> ("ILE CAN FRAMES"=→"ilosc mesagy":dbl, "Output CAN Array"=w266:string[][], "okres 100"=→"okres [ms]":dbl)  [unwired: 3 in, 2 out]
        "Frames" <- w266
        n125 = call "telemetria2.vi"("Input can Array"=w266) -> ("wiatr"=w250:T21, "temp/wilg"=w249:T22, "zap/kierunek"=w251:T23, "wyj nowe P"=→"wyj nowe P ? 2":cluster{"11":sgl, "12":sgl, "13":sgl}, "output cluster"=w253:T36, "wyj nowe L"=→"wyj nowe L ?":cluster{"8":sgl, "9":sgl, "10":sgl}, "ŚREDNIE NAPEDY"=→"srednie":T12, "MANIPULATOR wy"=→"MANIPULATOR wy" →"Wykres manipulator":T17, "pH"=w248:cluster{"temp. pkt rosy":sgl, "pH":sgl})  [unwired: 2 in]
        "RAW NAPEDY" <- w253
        "wiatr" <- w250
        "zap/kierunek" <- w251
        "temp/wilg" <- w249
        "pH" <- w248
        n126 = Bundle("zap/kierunek"=w251, "wiatr"=w250, "temp/wilg"=w249, "pH"=w248) -> (w247:T37)  [unwired: 1 in]
        n127 = call "Logger 2.vi"("output cluster"=w247, "RAW NAPEDY 2"=w253, "ON/OFF LOG"="LOG?", "path"="path") -> ()  [unwired: 8 in]
      }
      frame Error {
      }
    }
    "can" <- w244
  }
  "stope can" <- w12
  n128 = while {
    stop <- FALSE stop-if-true
    # "Wysyłanie do ROS-a"
    n129 = Wait Until Next ms Multiple(millisecond multiple=u32 1000 ("milliseconds to wait")) -> ()  [unwired: 1 out]
    n130 = case shown="True" "ROSB WRITE" {
      frame False {
      }
      frame True {
        n131 = TCP Open Connection(address="rosbridge server IP", remote port or service name="rosbridge port") -> (connection ID=w275:refnum<k5>, error out=w274:errorcluster)  [unwired: 3 in]
        n132 = TCP Write(connection ID=w275, data in="GET / HTTP/1.1\nUpgrade: websocket\nConnection: Upgrade\nHost: 192.168.5.103:9090\nOrigin: http://192.168.5.101:9090\nSec-WebSocket-Key: pM4mFvl5nUXJXjxIa41LvQ==\nSec-WebSocket-Version: 13", error in (no error)=w274) -> (connection ID out=w273:refnum<k5>, error out=w272:errorcluster)  [unwired: 1 in, 1 out]
        n133 = call <vilib>:"Write.vi"("error in (no error)"=w272, "Data"="advertise msg", "WebSocket Connection in"=w273) -> ("error out"=w290:errorcluster, "WebSocket Connection out"=w291:refnum<k5>)  [unwired: 7 in]
        n134 = while {
          tunnel: [w324] -> w283
          tunnel: [w323] -> w282
          tunnel: w291 -> [w325]
          tunnel: w290 -> [w326]
          stop <- "STOP ROS WRITE" stop-if-true
          w305 = -810.0
          w306 = 800.0
          # "m/s"
          # "obr/min"
          n135 = local read "srednie"() -> (w301:T12)
          n136 = Divide(x=w301, y=60.0 ("mean")) -> (x/y=w299:T12)
          n137 = Unbundle(w299) -> ("mean"=w309:dbl, "mean"=w308:dbl, "mean"=w307:dbl, "mean"=w302:dbl, "mean"=w303:dbl, "mean"=w304:dbl)
          n138 = Multiply(x=w302, y=w305) -> (x*y=w310:dbl)
          n139 = Multiply(x=w309, y=w306) -> (x*y=w313:dbl)
          n140 = Multiply(x=w303, y=w305) -> (x*y=w311:dbl)
          n141 = Multiply(x=w308, y=w306) -> (x*y=w314:dbl)
          n142 = Multiply(x=w304, y=w305) -> (x*y=w312:dbl)
          n143 = Multiply(x=w307, y=w306) -> (x*y=w315:dbl)
          n144 = To Word Integer(number=w311) -> (16bit integer=w293:i16)
          n145 = To Word Integer(number=w310) -> (16bit integer=w294:i16)
          n146 = To Word Integer(number=w312) -> (16bit integer=w292:i16)
          n147 = To Word Integer(number=w313) -> (16bit integer=w297:i16)
          n148 = To Word Integer(number=w315) -> (16bit integer=w295:i16)
          n149 = To Word Integer(number=w314) -> (16bit integer=w296:i16)
          n150 = Bundle By Name(cluster="szablon VELOCITIES", "op"="publish", "topic"="Topic to write", "msg.vel0"=w297, "msg.vel1"=w296, "msg.vel2"=w295, "msg.vel3"=w294, "msg.vel4"=w293, "msg.vel5"=w292) -> (w316:T1)
          n151 = Flatten To JSON(anything=w316, error in (no error)=w326) -> (JSON string=w320:string, 11:w322:errorcluster)  [unwired: 1 in]
          "raw frame" <- w320
          n152 = call <vilib>:"Write.vi"("error in (no error)"=w322, "Data"=w320, "WebSocket Connection in"=w325) -> ("error out"=w323:errorcluster, "WebSocket Connection out"=w324:refnum<k5>)  [unwired: 7 in]
          n153 = Wait (ms)(milliseconds to wait=u32 10) -> ()  [unwired: 1 out]
        }
        n154 = Search and Replace String(input string="advertise msg", search string="advertise", replace string="unadvertise" ("search string")) -> (result string=w278:string)  [unwired: 5 in, 3 out]
        n155 = call <vilib>:"Write.vi"("error in (no error)"=w282, "Data"=w278, "WebSocket Connection in"=w283) -> ("error out"=w284:errorcluster, "WebSocket Connection out"=w285:refnum<k5>)  [unwired: 7 in]
        n156 = call <vilib>:"Close.vi"("error in (no error)"=w284, "WebSocket Connection in"=w285) -> ("error out"=w288:errorcluster, "WebSocket Connection in"=w287:refnum<k5>)  [unwired: 8 in]
        n157 = TCP Close Connection(connection ID=w287, error in (no error)=w288) -> (error out=→"error out":errorcluster)  [unwired: 1 in, 1 out]
      }
    }
  }
  n158 = while {
    tunnel: [TRUE] -> w18
    tunnel: [w327] -> w15
    i -> [w329]
    stop <- w334 stop-if-true
    # "Lokalizacja"
    n159 = expression code="(x/180.0)*pi" "degrees to radians"("teta pocz.") -> (w331:dbl)
    n160 = Wait Until Next ms Multiple(millisecond multiple=u32 100) -> ()  [unwired: 1 out]
    n161 = while {
      shift-right: [w358] -> _
      shift-left: "Xo" -> [w345]
      shift-right: [w342] -> _
      shift-left: "Yo" -> [w343]
      shift-right: [w344] -> _
      shift-left: w331 -> [w359]
      tunnel: [TRUE] -> w327
      i -> [w338]
      stop <- w341 stop-if-true
      # "w"
      # "z"
      # "y"
      # "x"
      n162 = global read "Gobal for ROS.vi" "ROS read"() -> (w353:T38)
      n163 = Unbundle(w353) -> ("msg"=w354:T39)  [unwired: 2 out]
      n164 = call "Q to Euler.vi"("value"=w353) -> ("Yaw"=w352:dbl, "Waveform Chart"=→"pozycje z IMU":cluster{"Yaw":dbl, "Pitch":dbl, "Roll":dbl})  [unwired: 3 in, 2 out]
      "Yaw" <- w352
      n165 = local read "RAW NAPEDY"() -> (w336:T9)
      n166 = Unbundle(w354) -> ("axes"=w355:sgl[])  [unwired: 2 out]
      n167 = expression code="(x/180.0)*pi" "degrees to radians"(w352) -> ()  [unwired: 1 out]
      n168 = Wait Until Next ms Multiple(millisecond multiple=u32 50) -> ()  [unwired: 1 out]
      n169 = Index Array(array=w355) -> (element=w350:sgl)  [unwired: 1 in]
      n170 = call "Kinematyka_jazda.vi"("teta in"=w359, "RAW NAPEDY 2"=w336, "Yo"=w343, "Xo"=w345) -> ("po korekcie"=w344:dbl, "Y"=w342:dbl, "X"=w358:dbl, "teta"=→"teta":dbl)  [unwired: 4 in]
      "X" <- w358
      "Y" <- w342
      "po korekcie" <- w344
      n171 = Equal?(x=w350, y=sgl 1.0) -> (x = y?=→"obiekt?":bool)
      n172 = local read "stop all"() -> (w339:bool)
      n173 = disable-structure shown="Enabled" {
        frame Disabled {
          # "tło mapki"
          n174 = call <vilib>:"Read JPEG File.vi"("path to JPEG file"="path to JPEG file") -> ("image data"=w362:T40)  [unwired: 8 in, 2 out]
          n175 = call <vilib>:"Draw Flattened Pixmap.vi"("image data"=w362) -> ("new picture"=w363:picture)  [unwired: 8 in]
          n176 = property on="Location" class="XYGraph (strict)"("PlotImages.Back"=w363) -> ()  [unwired: 2 in, 2 out]
        }
        frame Enabled {
        }
      }
      n177 = Or(x="resset", y=w339) -> (x .or. y?=w341:bool)
      n178 = call "Build XY Graph"("Y Input"=w342, "X Input"=w358) -> ("XY Graph"=→"Location":cluster{"Y":dbl[], "Y":dbl[]}[])  [unwired: 8 in, 1 out]
      n179 = Greater?(x=w342, y="ile metrow ma przejechac ?") -> (0:→"przejechane ?":bool)
      "lok1" <- w338
    }
    n180 = local read "stop all"() -> (w334:bool)
    "lok" <- w329
  }
  "stope lokal" <- w18
  "stope lokal 2" <- w15
  n181 = while {
    tunnel: [w364] -> w14
    tunnel: w1 -> [w365]
    i -> [w367]
    stop <- w364 stop-if-true
    n182 = Wait Until Next ms Multiple(millisecond multiple=u32 1000 ("milliseconds to wait")) -> ()  [unwired: 1 out]
    n183 = case shown="True" "UDP from sb 2" {
      tunnel: w365 -> [_ w369]
      frame False {
      }
      frame True {
        w379 = 1000  # timeout ms
        w376 = 56 items=["No Error", "Argument Error", "Memory Full", "Out of Zone", "End of File", "File Already Open", "Generic File IO Error", "File Not Found", "File Permission Error", "Disk Full", "Duplicate Path", "Too Many Files Open", "Not Enabled", "Resource File Not Found", "Cannot Add Resource", "Resource Not Found", "Image Not Found", "Image Memory Error", "Pen Does Not Exist", "Config Bad Type", "Config Token Not Found", "Config Parse Error", "Config Memory Error", "Bad External Code Format", "Bad External Code Offset", "External Code Not Present", "Null Window", "Destroy Window Mixup", "Null Menu", "Print Aborted", "Bad Print Record", "Print Driver Error", "Windows Error During Print", "Memory Error During Print", "Print Dialog Error", "Generic Print Error", "Invalid Device Refnum", "Device Not Found", "Device Parameter Error", "Device Unit Error", "Can't Open Device", "Device Call Aborted", "Generic Error", "Cancelled By User", "Object ID Too Low", "Object ID Too High", "Object Not In Heap", "Unknown Heap", "Bad DefProc ID", "DefProc Not In Table", "Message Out Of Range", "Null Method", "Unknown Message", "Manager Call Not Supported", "Bad address", "Connection In progress", "Connection timed out", "Connection is already in progress", "Network attribute not supported", "Network error", "Address in use", "System out of memory", "Connection aborted", "Connection refused", "Connection is not connected", "Connection is already connected", "Connection closed", "Initialize error (interapplication manager)", "Bad occurrence", "Wait on unbound occurrence handler", "Occurrence queue overflow", "Bad path", "Semaphore not signaled", "Unrecognized type (interapplication manager)"] ("3rd Error to Convert")
        w377 = 62 items=["No Error", "Argument Error", "Memory Full", "Out of Zone", "End of File", "File Already Open", "Generic File IO Error", "File Not Found", "File Permission Error", "Disk Full", "Duplicate Path", "Too Many Files Open", "Not Enabled", "Resource File Not Found", "Cannot Add Resource", "Resource Not Found", "Image Not Found", "Image Memory Error", "Pen Does Not Exist", "Config Bad Type", "Config Token Not Found", "Config Parse Error", "Config Memory Error", "Bad External Code Format", "Bad External Code Offset", "External Code Not Present", "Null Window", "Destroy Window Mixup", "Null Menu", "Print Aborted", "Bad Print Record", "Print Driver Error", "Windows Error During Print", "Memory Error During Print", "Print Dialog Error", "Generic Print Error", "Invalid Device Refnum", "Device Not Found", "Device Parameter Error", "Device Unit Error", "Can't Open Device", "Device Call Aborted", "Generic Error", "Cancelled By User", "Object ID Too Low", "Object ID Too High", "Object Not In Heap", "Unknown Heap", "Bad DefProc ID", "DefProc Not In Table", "Message Out Of Range", "Null Method", "Unknown Message", "Manager Call Not Supported", "Bad address", "Connection In progress", "Connection timed out", "Connection is already in progress", "Network attribute not supported", "Network error", "Address in use", "System out of memory", "Connection aborted", "Connection refused", "Connection is not connected", "Connection is already connected", "Connection closed", "Initialize error (interapplication manager)", "Bad occurrence", "Wait on unbound occurrence handler", "Occurrence queue overflow", "Bad path", "Semaphore not signaled", "Unrecognized type (interapplication manager)"] ("1st Error to Convert")
        w371 = u16 61558  # port odbioru
        n184 = UDP Open(9:w379, 11:w371) -> (port=w372:refnum<k16>, 0:w373:errorcluster)  [unwired: 3 in, 1 out]
        n185 = while {
          tunnel: w372 -> [w385]
          tunnel: w373 -> [w386]
          tunnel: [w382] -> w374
          tunnel: [w381] -> w380
          tunnel: [w384] -> w370
          tunnel: w369 -> [w383]
          i -> [w388]
          stop <- "UDP odbior in" stop-if-true
          # "Odiór statusu z SBRIO"
          n186 = call "Odbiór UDP z SbRIO.vi"("Queue B in"=w383, "error in udp (no error)"=w386, "port"=w385) -> ("error out udp"=w381:errorcluster, "error out variant"=w384:errorcluster, "UDP Network Connection out"=w382:refnum<k16>)  [unwired: 6 in]
          n187 = Unbundle By Name(w381) -> ("status"=w389:bool)
          n188 = Not(x=w389) -> (.not. x?=→"UDP connection":bool)
          "receive ind" <- w388
        }
        n189 = UDP Close(connection ID=w374, 8:w380) -> (error out=w378:errorcluster)  [unwired: 1 out]
        n190 = call <vilib>:"Error to Warning.vi"("1st Error to Convert"=w377, "3rd Error to Convert"=w376, "error in"=w378) -> ("warning out"=w375:errorcluster)  [unwired: 3 in, 9 out]
        n191 = call <vilib>:"Simple Error Handler.vi"("error in (no error)"=w370) -> ()  [unwired: 1 in, 8 out]
        n192 = call <vilib>:"Simple Error Handler.vi"("error in (no error)"=w375) -> ()  [unwired: 1 in, 8 out]
      }
    }
    n193 = local read "stop all"() -> (w364:bool)
    "reciev lloop" <- w367
  }
  "stope odbior" <- w14
  n194 = while {
    tunnel: [w396] -> w25
    tunnel: [w391] -> w13
    tunnel: w4 -> [w394]
    i -> [w397]
    stop <- w391 stop-if-true
    n195 = call "Queue check.vi"("output cluster"=w394) -> ("output cluster 2"=w392:T29, "# elements in queue"=→"kolejka wysylanie":i32)  [unwired: 9 in]
    n196 = case shown="True" "UDP to sb 2" {
      tunnel: [w399 w402] -> w396
      tunnel: w392 -> [w400 w403]
      frame False {
        n197 = Unbundle By Name(w400) -> ("error out"=w399:errorcluster)
      }
      frame True {
        w406 = u16 58431  # lokalny port
        w409 = u16 58432  # port wysyłania
        w407 = "192.168.1.99"  # address
        w413 = 56 items=["No Error", "Argument Error", "Memory Full", "Out of Zone", "End of File", "File Already Open", "Generic File IO Error", "File Not Found", "File Permission Error", "Disk Full", "Duplicate Path", "Too Many Files Open", "Not Enabled", "Resource File Not Found", "Cannot Add Resource", "Resource Not Found", "Image Not Found", "Image Memory Error", "Pen Does Not Exist", "Config Bad Type", "Config Token Not Found", "Config Parse Error", "Config Memory Error", "Bad External Code Format", "Bad External Code Offset", "External Code Not Present", "Null Window", "Destroy Window Mixup", "Null Menu", "Print Aborted", "Bad Print Record", "Print Driver Error", "Windows Error During Print", "Memory Error During Print", "Print Dialog Error", "Generic Print Error", "Invalid Device Refnum", "Device Not Found", "Device Parameter Error", "Device Unit Error", "Can't Open Device", "Device Call Aborted", "Generic Error", "Cancelled By User", "Object ID Too Low", "Object ID Too High", "Object Not In Heap", "Unknown Heap", "Bad DefProc ID", "DefProc Not In Table", "Message Out Of Range", "Null Method", "Unknown Message", "Manager Call Not Supported", "Bad address", "Connection In progress", "Connection timed out", "Connection is already in progress", "Network attribute not supported", "Network error", "Address in use", "System out of memory", "Connection aborted", "Connection refused", "Connection is not connected", "Connection is already connected", "Connection closed", "Initialize error (interapplication manager)", "Bad occurrence", "Wait on unbound occurrence handler", "Occurrence queue overflow", "Bad path", "Semaphore not signaled", "Unrecognized type (interapplication manager)"] ("3rd Error to Convert")
        w414 = 62 items=["No Error", "Argument Error", "Memory Full", "Out of Zone", "End of File", "File Already Open", "Generic File IO Error", "File Not Found", "File Permission Error", "Disk Full", "Duplicate Path", "Too Many Files Open", "Not Enabled", "Resource File Not Found", "Cannot Add Resource", "Resource Not Found", "Image Not Found", "Image Memory Error", "Pen Does Not Exist", "Config Bad Type", "Config Token Not Found", "Config Parse Error", "Config Memory Error", "Bad External Code Format", "Bad External Code Offset", "External Code Not Present", "Null Window", "Destroy Window Mixup", "Null Menu", "Print Aborted", "Bad Print Record", "Print Driver Error", "Windows Error During Print", "Memory Error During Print", "Print Dialog Error", "Generic Print Error", "Invalid Device Refnum", "Device Not Found", "Device Parameter Error", "Device Unit Error", "Can't Open Device", "Device Call Aborted", "Generic Error", "Cancelled By User", "Object ID Too Low", "Object ID Too High", "Object Not In Heap", "Unknown Heap", "Bad DefProc ID", "DefProc Not In Table", "Message Out Of Range", "Null Method", "Unknown Message", "Manager Call Not Supported", "Bad address", "Connection In progress", "Connection timed out", "Connection is already in progress", "Network attribute not supported", "Network error", "Address in use", "System out of memory", "Connection aborted", "Connection refused", "Connection is not connected", "Connection is already connected", "Connection closed", "Initialize error (interapplication manager)", "Bad occurrence", "Wait on unbound occurrence handler", "Occurrence queue overflow", "Bad path", "Semaphore not signaled", "Unrecognized type (interapplication manager)"] ("1st Error to Convert")
        n198 = String To IP(1:w407) -> (0:w408:u32)
        n199 = UDP Open(11:w406) -> (port=w405:refnum<k16>, 0:w404:errorcluster)  [unwired: 4 in, 1 out]
        n200 = Bundle("port wysyłania"=w409, w408, "port"=w405, "error out"=w404) -> (w411:T41)  [unwired: 1 in]
        n201 = while {
          tunnel: [w424] -> w416
          tunnel: [w426] -> w410
          tunnel: w411 -> [w419]
          tunnel: w403 -> [w418]
          tunnel: [w417] -> w401
          i -> [w423]
          stop <- w422 stop-if-true
          # "Wysylanie  do SBRIO"
          n202 = call "Wysylanie UDP do SbRIO.vi"("Cluster"=w419, "output cluster"=w418) -> ("error out udp"=w424:errorcluster, "output cluster 2"=w417:T42, "connection ID out"=w426:refnum<k16>, "stop error ?"=w421:bool)  [unwired: 6 in]
          n203 = Wait (ms)(milliseconds to wait=u32 10) -> ()  [unwired: 1 out]
          n204 = Compound Arithmetic op=OR(w421, "udp to sbrio") -> (w422:bool)
          "send ind" <- w423
        }
        n205 = UDP Close(connection ID=w410, 8:w416) -> (error out=w415:errorcluster)  [unwired: 1 out]
        n206 = call "Queue destroy.vi"("output cluster"=w401) -> ("error out"=w402:errorcluster)  [unwired: 10 in]
        n207 = call <vilib>:"Error to Warning.vi"("1st Error to Convert"=w414, "3rd Error to Convert"=w413, "error in"=w415) -> ("warning out"=w412:errorcluster)  [unwired: 3 in, 9 out]
        n208 = call <vilib>:"Simple Error Handler.vi"("error in (no error)"=w412) -> ()  [unwired: 1 in, 8 out]
      }
    }
    n209 = Wait Until Next ms Multiple(millisecond multiple=u32 1000 ("milliseconds to wait")) -> ()  [unwired: 1 out]
    n210 = local read "stop all"() -> (w391:bool)
    "send loop" <- w397
  }
  "stope wysyl" <- w13
  n211 = while {
    tunnel: [w431] -> w10
    tunnel: [TRUE] -> w20
    i -> [w428]
    stop <- "stop all" stop-if-true
    w435 = u32 100  # millisecond multiple
    # "Safety and Health FPGA"
    n212 = shared-variable "NI-sbRIO9636-01A93195\\FPGA.lvlib\\temperatura"() -> (→"temperatura":sgl, error out=w430:errorcluster)  [unwired: 1 in]
    n213 = shared-variable "NI-sbRIO9636-01A93195\\FPGA.lvlib\\okres wg"("okres watchdoga", error in=w430) -> (error out=w432:errorcluster)
    n214 = shared-variable "NI-sbRIO9636-01A93195\\FPGA.lvlib\\wlacz watchdoga"("wlacz watchdoga", error in=w432) -> (error out=w431:errorcluster)
    n215 = Wait Until Next ms Multiple(millisecond multiple=w435) -> ()  [unwired: 1 out]
    "safety" <- w428
  }
  "stope health" <- w20
  n216 = while {
    tunnel: [TRUE] -> w19
    tunnel: w4 -> [w437]
    i -> [w439]
    stop <- w440 stop-if-true
    # "Obsługa przycisków"
    n217 = event shown="[1] Key Down;  Key Repeat" {
      selector: _ -> [_ _ _ _ _ _ _ _ _ _ _ _ _ _ _ _ _ _]
      dyn-events: _ -> [_ _ _ _ _ _ _ _ _ _ _ _ _ _ _ _ _ _]
      timeout: _ -> [_ _ _ _ _ _ _ _ _ _ _ _ _ _ _ _ _ _]
      tunnel: [_ _ _ _ _ TRUE _ _ _ _ _ _ _ _ _ _ _ _] -> w440
      tunnel: w437 -> [_ _ w471 w486 w504 _ w516 w518 _ w521 w524 w536 w545 w547 w570 w587 w590 w593]
      event Timeout {
        n218 = event-data() -> ()  [unwired: 1 in, 3 out]
      }
      event Key Down; Key Repeat {
        n219 = event-data() -> ("VKey"=w441:T45)  [unwired: 1 in]
        n220 = case shown="False" "klawiatura" {
          tunnel: w441 -> [_ w443]
          frame False {
          }
          frame True {
            n221 = case shown="\"Down\"" w443 {
              frame "ASCII", Default {
              }
              frame "Up" {
                n222 = local read "ster zadane"() -> (w449:cluster{dbl, dbl})
                n223 = Unbundle(w449) -> (w444:dbl, w448:dbl)
                n224 = Subtract(x=w444, y=sgl 1.0) -> (x-y=w446:dbl)
                n225 = Bundle(w446, w448) -> (w447:cluster{dbl, dbl})  [unwired: 1 in]
                n226 = local write "ster zadane"(w447) -> ()
              }
              frame "Down" {
                n227 = local read "ster zadane"() -> (w455:cluster{dbl, dbl})
                n228 = Unbundle(w455) -> (w450:dbl, w454:dbl)
                n229 = Add(x=w450, y=sgl 1.0) -> (x+y=w452:dbl)
                n230 = Bundle(w452, w454) -> (w453:cluster{dbl, dbl})  [unwired: 1 in]
                n231 = local write "ster zadane"(w453) -> ()
              }
              frame "Insert" {
                n232 = Bundle(0.0, 0.0) -> (w458:cluster{dbl, dbl})  [unwired: 1 in]
                n233 = local write "ster zadane"(w458) -> ()
              }
              frame "Left" {
                n234 = local read "ster zadane"() -> (w464:cluster{dbl, dbl})
                n235 = Unbundle(w464) -> (w459:dbl, w461:dbl)
                n236 = Subtract(x=w461, y=sgl 1.0) -> (x-y=w462:dbl)
                n237 = Bundle(w459, w462) -> (w463:cluster{dbl, dbl})  [unwired: 1 in]
                n238 = local write "ster zadane"(w463) -> ()
              }
              frame "Right" {
                n239 = local read "ster zadane"() -> (w470:cluster{dbl, dbl})
                n240 = Unbundle(w470) -> (w467:dbl, w466:dbl)
                n241 = Add(x=w466, y=sgl 1.0) -> (x+y=w468:dbl)
                n242 = Bundle(w467, w468) -> (w469:cluster{dbl, dbl})  [unwired: 1 in]
                n243 = local write "ster zadane"(w469) -> ()
              }
            }
          }
        }
      }
      event "Prędkosci Prawy [4]": Value Change {
        w474 = u32 0 ("identifier")
        n244 = event-data() -> ()  [unwired: 1 in, 6 out]
        n245 = Select(t=u8 1 ("identifier"), s="Prędkosci Prawy [4]", f=u8 0 ("identifier")) -> (s? t:f=w476:u8)
        n246 = Build Array(u32 5 ("identifier"), w476, w474, w474, w474, w474, w474, w474) -> (w480:u32[])
        n247 = Bundle By Name(cluster=T30 {"identifier"=0, "extended?"=FALSE, "type"=0, "payload"=[]} ("CAN frame 2"), "payload"=w480, "identifier"=u32 1) -> (w485:T30)
        n248 = To Variant(anything=w485) -> (Variant=w482:variant)
        n249 = Bundle By Name(cluster=T28 {"Message"="", "Message Data"=variant} ("Message Cluster"), "Message"="4", "Message Data"=w482) -> (w472:T28)
        n250 = call "Queue add.vi"("Queue B in"=w471, "Message Cluster"=w472) -> ()  [unwired: 10 in]
      }
      event "Prędkości Lewy [5]": Value Change {
        w490 = u32 0 ("identifier")
        n251 = event-data() -> ()  [unwired: 1 in, 6 out]
        n252 = Select(t=u8 1 ("identifier"), s="Prędkości Lewy [5]", f=u8 0 ("identifier")) -> (s? t:f=w492:u8)
        n253 = Build Array(u32 5 ("identifier"), w492, w490, w490, w490, w490, w490, w490) -> (w495:u32[])
        n254 = Bundle By Name(cluster=T30 {"identifier"=0, "extended?"=FALSE, "type"=0, "payload"=[]} ("CAN frame 2"), "payload"=w495, "identifier"=u32 2) -> (w500:T30)
        n255 = To Variant(anything=w500) -> (Variant=w497:variant)
        n256 = Bundle By Name(cluster=T28 {"Message"="", "Message Data"=variant} ("Message Cluster"), "Message"="4", "Message Data"=w497) -> (w487:T28)
        n257 = call "Queue add.vi"("Queue B in"=w486, "Message Cluster"=w487) -> ()  [unwired: 10 in]
      }
      event "manipulator [32]": Value Change {
        w503 = u32 0 ("identifier")
        n258 = event-data() -> ()  [unwired: 1 in, 6 out]
        n259 = Select(t=u8 254 ("identifier"), s="manipulator [32]", f=u8 255 ("identifier")) -> (s? t:f=w502:u8)
        n260 = Build Array(w502, w503, w503, w503, w503, w503, w503, w503) -> (w509:u32[])
        n261 = Bundle By Name(cluster=T30 {"identifier"=0, "extended?"=FALSE, "type"=0, "payload"=[]} ("CAN frame 2"), "payload"=w509, "identifier"=u32 3) -> (w514:T30)
        n262 = To Variant(anything=w514) -> (Variant=w511:variant)
        n263 = Bundle By Name(cluster=T28 {"Message"="", "Message Data"=variant} ("Message Cluster"), "Message"="4", "Message Data"=w511) -> (w505:T28)
        n264 = call "Queue add.vi"("Queue B in"=w504, "Message Cluster"=w505) -> ()  [unwired: 10 in]
      }
      event "eventy stop": Value Change {
        n265 = event-data() -> ()  [unwired: 1 in, 6 out]
      }
      event "stop queue": Value Change {
        n266 = event-data() -> ()  [unwired: 1 in, 6 out]
        n267 = call "Queue add.vi"("Queue B in"=w516, "Message Cluster"=T28 {"Message"="Exit", "Message Data"=variant} ("element")) -> ()  [unwired: 10 in]
      }
      event Value Change {
        n268 = event-data() -> ()  [unwired: 1 in, 6 out]
        n269 = call "PrzódL.vi"("Konfiguracja"="PRZOD P") -> ("Message Cluster"=w519:T28)  [unwired: 10 in]
        n270 = call "Queue add.vi"("Queue B in"=w518, "Message Cluster"=w519) -> ()  [unwired: 10 in]
      }
      event "E-Stop": Value Change {
        n271 = event-data() -> ()  [unwired: 1 in, 6 out]
      }
      event Value Change {
        n272 = event-data() -> ()  [unwired: 1 in, 6 out]
        n273 = call "PrzódL.vi"("Konfiguracja"="SRODEK P") -> ("Message Cluster"=w522:T28)  [unwired: 10 in]
        n274 = call "Queue add.vi"("Queue B in"=w521, "Message Cluster"=w522) -> ()  [unwired: 10 in]
      }
      event Value Change {
        n275 = event-data() -> ()  [unwired: 1 in, 6 out]
        n276 = call "PrzódL.vi"("Konfiguracja"="TYL P") -> ("Message Cluster"=w525:T28)  [unwired: 10 in]
        n277 = call "Queue add.vi"("Queue B in"=w524, "Message Cluster"=w525) -> ()  [unwired: 10 in]
      }
      event "PITCH 1", "YAW 1", "ROLL 1": Value Change {
        n278 = event-data() -> ()  [unwired: 1 in, 6 out]
        n279 = Bundle By Name(cluster=T43 {"PITCH 1"=0.0, "YAW 1"=0.0, "ROLL 1"=0.0} ("Gimbale"), "PITCH 1"="PITCH 1", "YAW 1"="YAW 1", "ROLL 1"="ROLL 1") -> (w527:T43)
        n280 = To Variant(anything=w527) -> (Variant=w530:variant)
        n281 = Bundle By Name(cluster=T28 {"Message"="", "Message Data"=variant} ("Message Cluster"), "Message"="5", "Message Data"=w530) -> (w528:T28)
        n282 = call "Queue add.vi"("Queue B in"=w536, "Message Cluster"=w528) -> ()  [unwired: 10 in]
      }
      event "STOP ??", "RESET STM": Value Change {
        n283 = event-data() -> ()  [unwired: 1 in, 6 out]
        n284 = Bundle By Name(cluster=T44 {"reset_stm"=TRUE, "stop"=TRUE} ("safety ctl"), "stop"="STOP ??", "reset_stm"="RESET STM") -> (w539:T44)
        n285 = To Variant(anything=w539) -> (Variant=w542:variant)
        n286 = Bundle By Name(cluster=T28 {"Message"="", "Message Data"=variant} ("Message Cluster"), "Message"="6", "Message Data"=w542) -> (w540:T28)
        n287 = call "Queue add.vi"("Queue B in"=w545, "Message Cluster"=w540) -> ()  [unwired: 10 in]
      }
      event "Stop wózek", "Wózek up", "Wózek down", "Wózek PWM", "Stop głębokość", "Gkebokość PWM", "Wiertło PWM", "ON/OFF Wiertło", "SERWO 4", "SERWO 5", "pojrmniki 6", "chwytak 3": Value Change {
        n288 = event-data() -> ()  [unwired: 1 in, 5 out]
        n289 = Bundle("pojrmniki 6"="pojrmniki 6", "SERWO 5"="SERWO 5", "SERWO 4"="SERWO 4", "chwytak 3"="chwytak 3", "ON/OFF Wiertło"="ON/OFF Wiertło", "Wiertło PWM"="Wiertło PWM", "Gkebokość PWM"="Gkebokość PWM", "Stop głębokość"="Stop głębokość", "Wózek PWM"="Wózek PWM", "speed wózek"="speed wózek", "Wózek up"="Wózek up", "Wózek down"="Wózek down", "Stop wózek"="Stop wózek", "PROBNK ID 4"="PROBNK ID 4") -> (w548:T46)  [unwired: 1 in]
        "kluster sterowan probnik" <- w548
        n290 = call "próbnik.vi"("output cluster 2"=w548) -> ("Message Cluster"=w559:T28, "number stopy"=w553:u32)  [unwired: 9 in]
        n291 = call "Queue add.vi"("Queue B in"=w547, "Message Cluster"=w559) -> ()  [unwired: 10 in]
        n292 = case shown="1" w553 {
          frame 2, 3 {
            n293 = property on="Gkebokość PWM" class="Slide (strict)"("Value"=u8 128 ("Wózek PWM")) -> ()  [unwired: 2 in, 2 out]
          }
          frame 0, Default {
            n294 = property on="Wiertło PWM" class="Slide (strict)"("Value"=u8 128 ("Wózek PWM")) -> ()  [unwired: 2 in, 2 out]
          }
          frame 1 {
          }
          frame 4, 5 {
            n295 = property on="Wózek PWM" class="Slide (strict)"("Value"=u8 128 ("Wózek PWM")) -> ()  [unwired: 2 in, 2 out]
          }
        }
      }
      event "Zbiornik", "Stop zbiorniki", "Zbiornik 2", "Stop zbiorniki 2": Value Change {
        w571 = u8 0 ("identifier")
        n296 = event-data() -> ()  [unwired: 1 in, 6 out]
        n297 = case shown="True" "Stop zbiorniki 2" {
          tunnel: [w583 w584] -> w567
          tunnel: "Zbiornik 2" -> [w583 _]
          frame False {
          }
          frame True {
            w584 = u8 128 ("identifier")
            n298 = property on="Zbiornik 2" class="Slide (strict)"("Value"=w584) -> ()  [unwired: 2 in, 2 out]
          }
        }
        n299 = case shown="True" "Stop zbiorniki" {
          tunnel: [w585 w586] -> w572
          tunnel: "Zbiornik" -> [w585 _]
          frame False {
          }
          frame True {
            w586 = u8 128 ("identifier")
            n300 = property on="Zbiornik" class="Slide (strict)"("Value"=w586) -> ()  [unwired: 2 in, 2 out]
          }
        }
        n301 = Build Array(w572, w567, w571, w571, w571, w571, w571, w571) -> (w580:u8[])
        n302 = Bundle By Name(cluster=T30 {"identifier"=0, "extended?"=FALSE, "type"=0, "payload"=[]} ("CAN frame 2"), "payload"=w580, "identifier"=u32 5) -> (w575:T30)
        n303 = To Variant(anything=w575) -> (Variant=w578:variant)
        n304 = Bundle By Name(cluster=T28 {"Message"="", "Message Data"=variant} ("Message Cluster"), "Message"="3", "Message Data"=w578) -> (w582:T28)
        n305 = call "Queue add.vi"("Queue B in"=w570, "Message Cluster"=w582) -> ()  [unwired: 10 in]
      }
      event Value Change {
        n306 = event-data() -> ()  [unwired: 1 in, 6 out]
        n307 = call "PrzódL.vi"("Konfiguracja"="PRZOD L") -> ("Message Cluster"=w588:T28)  [unwired: 10 in]
        n308 = call "Queue add.vi"("Queue B in"=w587, "Message Cluster"=w588) -> ()  [unwired: 10 in]
      }
      event Value Change {
        n309 = event-data() -> ()  [unwired: 1 in, 6 out]
        n310 = call "PrzódL.vi"("Konfiguracja"="TYL L") -> ("Message Cluster"=w591:T28)  [unwired: 10 in]
        n311 = call "Queue add.vi"("Queue B in"=w590, "Message Cluster"=w591) -> ()  [unwired: 10 in]
      }
      event Value Change {
        n312 = event-data() -> ()  [unwired: 1 in, 6 out]
        n313 = call "PrzódL.vi"("Konfiguracja"="SRODEK L") -> ("Message Cluster"=w594:T28)  [unwired: 10 in]
        n314 = call "Queue add.vi"("Queue B in"=w593, "Message Cluster"=w594) -> ()  [unwired: 10 in]
      }
    }
    "eventy ind" <- w439
  }
  "stope event" <- w19
  n315 = Merge Errors(w10) -> (w11:errorcluster)
  n316 = call-poly <vilib>:"Close Input Device.vi"("error in (no error)"=w30, "device ID"=w31) -> ("error out"=w9:errorcluster)  [unwired: 8 in]
  n317 = call-poly <vilib>:"Close Input Device.vi"("error in (no error)"=w28, "device ID"=w29) -> ("error out"=w7:errorcluster)  [unwired: 8 in]
  n318 = Merge Errors(w11) -> (w8:errorcluster)
  n319 = disable-structure shown="Disabled" {
    disable-tunnel: [w600 _] -> _
    disable-tunnel: [w599 _] -> _
    disable-tunnel: [w598 _] -> _
    disable-tunnel: _ -> [w597 _]
    disable-tunnel: _ -> [w596 _]
    frame Disabled {
      n320 = call "ROSBRIDGE TCP READ.vi"("error in (no error)"=w596, "String in"="", "TCP Network Connection in"=w597) -> ("error out"=w598:errorcluster, "String out"=w600:string, "TCP Network Connection out"=w599:refnum<k5>)  [unwired: 6 in]
    }
    frame Enabled {
    }
  }
  n321 = Merge Errors(w8, w9) -> (w6:errorcluster)
  n322 = Merge Errors(w6, w7, w25) -> (w26:errorcluster)
  n323 = call <vilib>:"Simple Error Handler.vi"("error in (no error)"=w26) -> ()  [unwired: 1 in, 8 out]
